vi "UHR-Fleezers Control (fpga) - 11.7.1UCBMeng3RG3(2).vi"() -> ()   [LabVIEW 2014]
doc: "UHR-Fleezers Instrument Control Code (fpga)"
uses:
  <vilib>/Platform/TimedLoop/XDataNode/timing_clust.ctl
  <vilib>/Platform/TimedLoop/XDataNode/nitl_modes.ctl
  <vilib>/Platform/TimedLoop/XDataNode/wakeup.ctl
  <vilib>/rvi/Emulation/niFpgaGetClockAttributes.vi
  <vilib>/rvi/Emulation/niFpgaSctlEmulationGetInTimedLoop.vi
  <vilib>/rvi/Emulation/niFpgaEmulationReportErrorSimple.vi
  <vilib>/rvi/Emulation/niFpgaProcessEmulError.vi
  <vilib>/rvi/eio/common/nirviEmuTemplateMethod_errors.vi
  <vilib>/rvi/Emulation/niFpgaCriticalErrorInLSC.vi
  <vilib>/rvi/interface/RandomDataEmulation/niFpgaRandomDataHandleErrors.vi
  <vilib>/eio/EIONode/EIONode.xnode
  <vilib>/eio/EIOMethodNode/EIOMethodNode.xnode
  <vilib>/rvi/DataTransferAndStorage/Container/XNode/niFpgaContainer.xnode
  <vilib>/rvi/interface/RandomDataEmulation/nirviRandomDataFpgaReadWriteTemplate.vi
  <vilib>/addons/control/pid/fpga.llb/XNode/niFpgaPID.xnode
  <vilib>/Platform/TimedLoop/XDataNode/XDataNode.xnode
  <vilib>/Platform/TimedLoop/XDataNode/XDNodeRunTimeDep.lvlib
panel:
  in  "Tab Control":T1(tab)=enum."Force FB"
  in  "Set 3":bool
  in  "Set 2":bool=TRUE
  in  "Set 1":bool=TRUE
  in  "Trap Pos to FIFO":bool
  in  "N of AI1 Int Acq Sets":i16=2 min=1 max=3 step=1
  out "AI Late Counter":u8
  in  "ai count":u16=400
  in  "+ phase":bool
  in  "Phase count adjustment":i16
  out "Relative phase":i16
  in  "AI to FIFO":bool
  out "BD1 Frequency Out 1":u64
  out "BD1 Frequency Out 2":u64
  out "Trap Pos FIFO Timeout":u16
  out "Trap AI FIFO Timeout":u16
  in  "Trap FIFO Set Timeout":i32
  in  "Tab Control 2":T2(tab)
  in  "FB Offset":u16
  in  "FB Multi Factor":i16
  in  "Dynamic FB (Ronen)":bool
  in  "Negate Intensity FB":bool
  in  "RD":bool
  in  "FB1 output high":i16=3000
  in  "FB1 output low":i16
  in  "D1":i16
  in  "I1":i16=5
  in  "P1":i16=10
  in  "Swap F1 and F2":bool
  in  "Cont. Scan":bool
  in  "Abort scan":bool
  in  "Cycles per step":u64
  in  "Scan BD":bool
  in  "Number of scans":u16
  in  "Scan steps":u64
  in  "Scan freq.  increment":i64
  out "Scanning":bool
  in  "Start scan":bool
  in  "OSK Bd 1":bool
  in  "Reset Bd 1":bool
  in  "PMODE":bool
  in  "Direct RF Box \nCommunication":bool
  in  "Data BD 2":u8 format="%08b"
  in  "Data BD 1":u8 format="%08b"
  in  "Address":u8 format="%02x"
  in  "Update Data":bool
  in  "FPGA Controls\n RF Box":bool
  in  "Number Interlace Cycles":u8=2 min=1 max=3
  in  "Interlace Off Parameters":u8=1 min=1 max=3
  in  "Interlace ON/OFF":bool
  out "DIO Relative phase":i16
  in  "Phase count adjustment (DIO)":i16
  in  "+ phase (DIO)":bool
  out "DIO Late Counter":u8
  in  "DIO count 1 (ticks)":u16=400
  in  "DIO count 2 (ticks)":u16=400
  in  "DIO count 3 (ticks)":u16=400
  out "AI2 Y Sum Set 2":i16
  out "AI2 Y Sum Set 1":i16
  in  "FB Setpoint Set 1":i16 min=0 step=1
  in  "FB Reset Set 1":bool
  in  "FB On/Off Set 1":bool
  in  "FB Reset Set 2":bool
  in  "FB On/Off Set 2":bool
  in  "FB Setpoint Set 2":i16 min=0 step=1
  out "Scan I":u64
  in  "Amp switch delay":u8=5
  in  "XY phase ext loop method":bool
  in  "BD 2 Amplitude 1":u16
  in  "BD 1 Amplitude 1":u16
  in  "BD 2 Frequency 1":u64
  in  "BD 1 Frequency 1":u64
  in  "BD 2 Amplitude 2":u16
  in  "BD 1 Amplitude 2":u16
  in  "BD 2 Frequency 2":u64
  in  "BD 1 Frequency 2":u64
  in  "BD 2 Amplitude 3":u16
  in  "BD 1 Amplitude 3":u16
  in  "BD 2 Frequency 3":u64
  in  "BD 1 Frequency 3":u64
  in  "BD 1 Delay (ticks)":u8
  in  "BD 2 Delay (Ticks)":u8 caption="Count(Ticks)"
  in  "Next trap write delay (ticks)":u8 caption="Count(Ticks)"
  in  "Trap 1 osc enable":bool
  in  "Trap 2 osc enable":bool
  in  "FB Min frequency":u64
  in  "FB Max Frequency":u64
  in  "Dynamic Force FB (Ronen)":bool
  in  "FB2 output high":fxp<+/-,16,1>=0.999969482421875
  in  "FB2 output low":fxp<+/-,16,1>=-1.0
  in  "P2":fxp<+/-,16,8> format="%.11g"
  in  "I2":fxp<+/-,16,8>=10.0 format="%.11g"
  in  "D2":fxp<+/-,16,8> format="%.11g"
  in  "Negate Diff?":bool
  in  "Diff FB Measurement?":bool
  in  "FB Trig Integrate":u32=1
  out "TTrig?":bool
  in  "TTrig Negate Pos":bool=TRUE
  out "Trap Pos FB Int Signal":fxp<+/-,24,9> format="%.18g"
  out "Trap Pos FB Int-Norm Signal":fxp<+/-,16,1> format="%.16g"
  in  "FPGA TTrig Thresh":i64
  in  "FPGA Trap Trig":bool
  out "Trap Pos FB Action":i64
  in  "Trap Pos. FB Offset Factor":i64
  in  "Trap Pos. FB Mult Factor":i64=2
  in  "Trap Pos. FB Reset":bool
  in  "Trap Pos FB Monitor T1 or T2":bool
  in  "AI1 X Scale":u16
  in  "Trap Pos FB Int Count":u16=100
  in  "Trap Pos FB Negate Action":bool
  out "AI1 X Set 2":fxp<+/-,16,1>
  out "AI1 X Set 1":fxp<+/-,16,1>
  in  "Trap Pos. FB SP":fxp<+/-,16,1>
  in  "Force feedback":bool
  out "TTrig Sig":i64
  out "TTrig Fin Thresh":i64
  in  "1D or 2D Scan?":bool
  in  "Abort scan (MCL)":bool
  in  "MCL Scan Axis":bool
  in  "Cont. Scan (MCL)":bool
  out "Scan I (MCL)":u64
  in  "Number of scans (MCL)":u16
  out "Scanning MCL":bool
  in  "Scan steps (MCL)":u64
  in  "Cycles per step (MCL)":u64
  in  "Scan freq.  increment (MCL)":i16
  in  "Start scan (MCL)":bool
  in  "AO2":i16
  in  "AO1":i16
  out "MCL Late Counter":u8
  in  "MCL count":u32=800
  out "MCL Relative Phase":i16
  in  "Phase count adjustment (MCL)":i16
  in  "+ phase (MCL)":bool
  out "APD2 int gate":bool
  out "APD3 out state":bool
  in  "APD Gate Operating Mode":u8 max=2 step=1
  in  "Invert APD Gate":bool
  in  "APD Gate OFF Count":u16=100
  in  "APD Gate ON Count":u16=300
  out "APD 1 Gate Late Counter":u8
  out "APD 1 Gate Relative Phase":i16
  in  "Phase count adjustment (APD 1 Gate)":i16
  in  "+ phase (APD 1 Gate)":bool
  out "APD 2 Counts 0":u32
  out "APD 2 Counts 1":u32
  out "APD 1 Counts 0":u32
  out "APD 1 Counts 1":u32
  out "APD1 out state":bool
  in  "APD AO scale factor":i16=1
  in  "APD to FIFO":bool
  in  "APD Acq Rate Count":u32=20000000
  out "APD Acq Late Counter":u8
  out "APD Acq Relative Phase":i16
  in  "Phase Count Adjustment (APD Acq)":i16
  in  "+ phase (APD Acq)":bool
  in  "Phase count adjustment (APD 2 Gate)":i16
  out "APD 2 Gate Late Counter":u8
  out "APD 2 Gate Relative Phase":i16
  in  "+ phase (APD 2 Gate)":bool
  out "APD2 out state":bool
  out "APD 3 Counts 0":u32
  out "APD 3 Counts 1":u32
  out "APD 3 Gate Late Counter":u8
  in  "Phase count adjustment (APD 3 Gate)":i16
  out "APD 3 Gate Relative Phase":i16
  in  "+ phase (APD 3 Gate)":bool
  out "APD1 int gate":bool
  out "APD3 int gate":bool
  in  "D3":i16
  in  "I3":i16=5
  in  "P3":i16=10
  in  "Green Filter Flipper":bool
  in  "Green FB Count":u16=1200
  out "Green Late Counter":u8
  out "Green FB Relative Phase":i16
  in  "Phase count adjustment (Green FB)":i16=10
  in  "+ phase (Green FB)":bool
  out "Green FB Sum":i16
  in  "Green int current ON count adj":u16=150
  in  "Current Out":u16=30000
  in  "Green FB On/Off":bool
  in  "Green FB Setpoint":i16=250 min=0 step=1
  in  "Green FB Reset":bool
  in  "Operating Mode 2":u8=2 max=2 step=1
  in  "Invert GI 2":bool
  in  "Green interlace OFF count 2":u16=900
  in  "Green interlace ON count 2":u16=300
  out "GI Late Counter 2":u8
  out "GI Relative phase 2":i16
  in  "Phase count adjustment (GI) 2":i16=20
  in  "+ phase (GI) 2":bool
  in  "Green interlace OFF count":u16=100
  out "GI Relative phase":i16
  in  "Phase count adjustment (GI)":i16
  in  "+ phase (GI)":bool
  in  "Green interlace ON count":u16=300
  out "GI Late Counter":u8
  in  "Invert GI":bool
  in  "Operating Mode":u8 max=2 step=1
  in  "+ phase (RI)":bool
  out "RI Relative phase":i16
  out "RI Late Counter":u8
  in  "Red interlace ON count":u16=300
  in  "Red interlace OFF count":u16=100
  in  "Invert RI":bool
  in  "Red Laser Operating Mode":u8 max=2 step=1
  in  "Phase count adjustment (RI)":i16
  out "Red FB Intensity":i16
  in  "RI Current Out":u16=30000
  in  "Red FB On/Off":bool
  in  "D4":i16
  in  "I4":i16=5
  in  "P4":i16=10
  in  "Red FB Setpoint":i16=250 min=0 step=1
  in  "Red FB Reset":bool
  in  "RI Operating Mode 2":u8=2 max=2 step=1
  in  "Invert RI 2":bool
  in  "Phase count adjustment (BI AO)":i16=20
  in  "Blue current ON count adj (AO)":u16=150
  in  "BI Current Out":i16=30000
  in  "Blue FB On/Off":bool
  in  "D5":i16
  in  "I5":i16=5
  in  "P5":i16=10
  in  "Blue FB Setpoint":i16=250 min=0 step=1
  in  "Blue FB Reset":bool
  in  "BI Operating Mode (AO)":u8=2 max=2 step=1
  in  "Invert BI (AO)":bool
  in  "Blue OFF count (AO)":u16=900
  in  "Blue ON count (AO)":u16=300
  out "BI Late Counter (AO)":u8
  out "BI Relative phase (AO)":i16
  in  "+ phase (BI AO)":bool
  in  "Phase count adjustment (BI D)":i16
  in  "Blue Laser Operating Mode (D)":u8 max=2 step=1
  in  "Invert BI (D)":bool
  in  "Blue interlace OFF count (D)":u16=100
  in  "Blue interlace ON count (D)":u16=300
  out "Blue Late Counter (D)":u8
  out "BI Relative phase (D)":i16
  in  "+ phase (BI D)":bool
  out "Blue Intensity":i16
  # "Only one of these can be on\nat a time:"
  # "Raster Scan AOD"
  # "1 (X)"
  # "2 (Y)"
  # "IR Intensity Feedback (RF BD 1)"
  # "FB Gains Set 1"
  # "FB output range 1"
  # "False is usual, True is external loop method"
  # "Parameters if using the external RF switching loop"
  # "Parameters if using the usual internal RF switching method"
  # "FB Triggering Excitation Laser"
  # "Trap Pos. FB Gains"
  # "Trap Pos. FB Range"
  # "AO1 (Y)"
  # "2D"
  # "1D"
  # "AO2 (X)"
  # "APD AO for aligning"
  # "Detection Loop"
  # "Green fluorescent laser digital gate interlacing loop"
  # "0 Forced ON\n1 Forced OFF\n2 Interlacing"
  # "Green FB Gains"
  # "Red fluorescent laser digital gate interlacing loop"
  # "Detection Loop"
  # "0 Forced ON\n1 Forced OFF\n2 Interlacing"
  # "Analog/FB Control Loop\n(Disabled)"
  # "Digital Control Loop"
  # "Blue laser intensity reading"
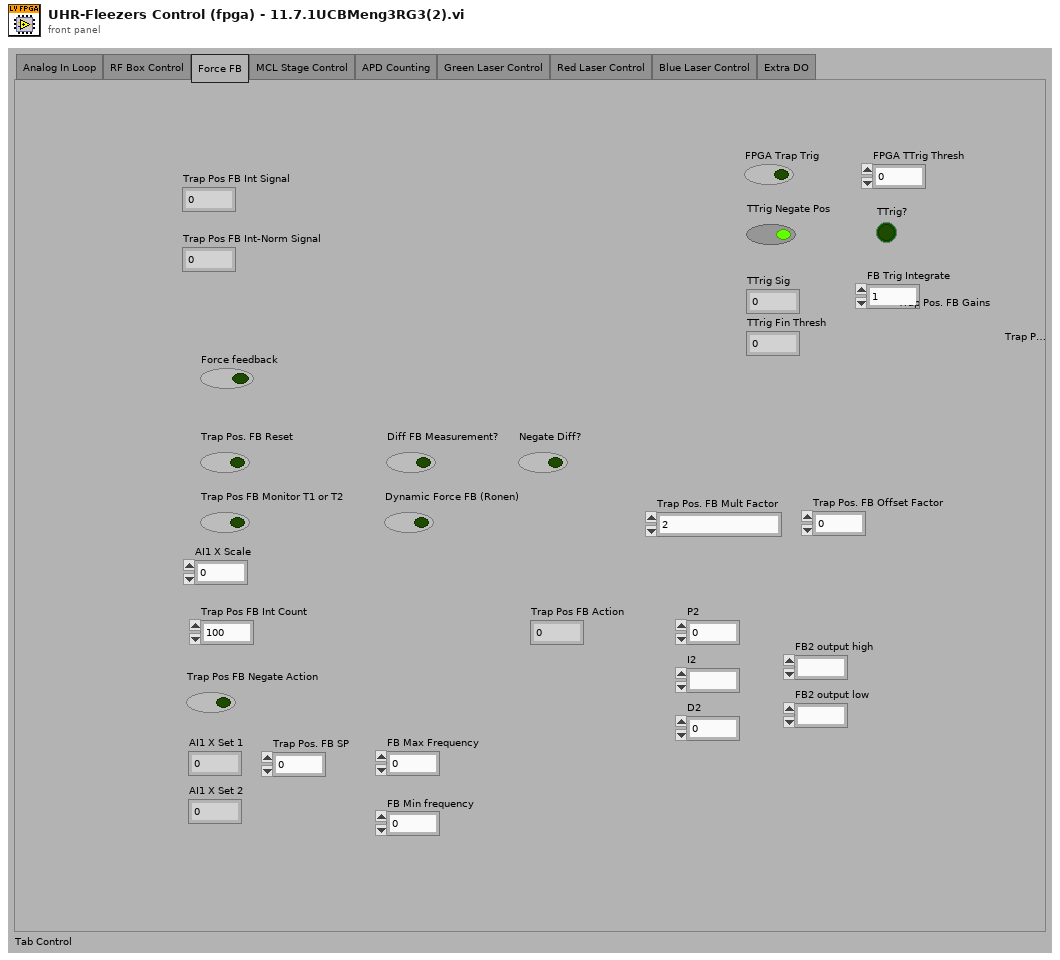
[diagram p1: front panel]
types:
  T1 = enum32{"Analog In Loop", "RF Box Control", "Force FB", "MCL Stage Control", "APD Counting", "Green Laser Control", "Red Laser Control", "Blue Laser Control", "Extra DO"}
  T2 = enum32{"Controls", "Interlacing Frequency and Amplitude Values", "Oscillate trap from memory"}
  T3 = typedef "XDNodeRunTimeDep.lvlib/timing_clust.ctl" = cluster{"Expected End [f-1]":u64, "Actual End [f-1]":u64, "Finished Late? [f-1]":bool, "Expected End [i-1]":u64, "Actual End [i-1]":u64, "Finished Late? [i-1]":bool, "Expected Start [i]":u64, "Actual Start [i]":u64, "Expected Start [f]":u64, "Actual Start [f]":u64, "Source Name":string, "Structure Name":string, "Period":i64, "Deadline":i64, "Offset":i64, "Start":i64, "Priority":i32, "Timeout":i32, "Mode":T4, "Wakeup Reason":T5, "Error":errorcluster, "Source Type":string, "Secondary Source Type":string, "Global End Time":u64, "Global Start Time":u64, "Frame Duration":u64, "Iteration Duration":u64, "Assigned CPU":i32, "I/O Scan Engine Mode":u32}
  T4 = typedef "XDNodeRunTimeDep.lvlib/nitl_modes.ctl" = enum32{"No Change", "Process missed periods, maintain original phase", "Discard missed periods, maintain original phase", "Process missed periods, ignore original phase", "Discard missed periods, ignore original phase"}
  T5 = typedef "XDNodeRunTimeDep.lvlib/wakeup.ctl" = enum32{"Normal", "Aborted", "Asynchronous wakeup", "Timing source error", "Timed loop error", "Timeout"}
  T6 = cluster{"proportional gain (Kc)":i16, "integral gain (Kc*Ts/Ti)":i16, "derivative gain (Kc*Td/Ts)":i16}
  T7 = cluster{"FB1 output high":i16, "FB1 output low":i16}
  T8 = cluster{"P2":fxp<+/-,16,8>, "I2":fxp<+/-,16,8>, "D2":fxp<+/-,16,8>}
  T9 = cluster{"FB2 output high":fxp<+/-,16,1>, "FB2 output low":fxp<+/-,16,1>}
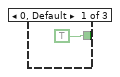
[diagram p2: hidden frame]
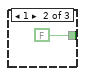
[diagram p3: hidden frame]
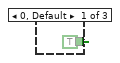
[diagram p4: hidden frame]
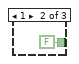
[diagram p5: hidden frame]
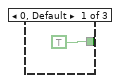
[diagram p7: hidden frame]
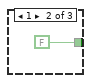
[diagram p8: hidden frame]
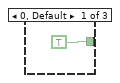
[diagram p10: hidden frame]
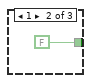
[diagram p11: hidden frame]
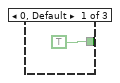
[diagram p14: hidden frame]
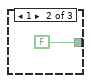
[diagram p15: hidden frame]
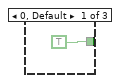
[diagram p17: hidden frame]
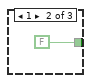
[diagram p18: hidden frame]
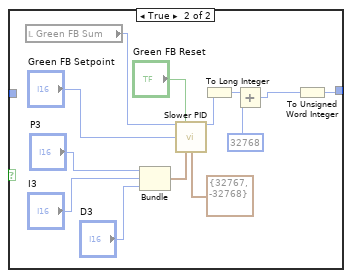
[diagram p20: hidden frame]
diagram:
  w7 = FALSE
  w5 = FALSE
  # "timing array current index"
  # "timing array"
  # "timing counter (phase adjusted here)"
  # "late counter"
  n1 = flat-sequence "FPGA initialization to do before running any of the loops" {
    tunnel: [u16 0 ("DIO count 3 (ticks)")] -> w4
    tunnel: [w15] -> _
    frame #0 {
      w14 = FALSE ("Enable")
      # "BD 2 (Y)"
      # "BD 1 (X)"
      # "Start up expansion chassis early\nto avoid delays later"
      # "This pin controls udclk on the RF boards.\nWhen initially configuring the boards, this pin needs to be\nconfigured as a high impedance input.  Later it will be switched\nto an output."
      # "Initial setting of DIO data and \naddress to low (before reset).  \nThis needs to happen before the other\ncontrol method loops execute."
      n2 = xnode "FPGA I/O Node"("Chassis2/Mod1/AO0"=u16 0 ("Chassis2/Mod4/AO0")) -> ("Chassis2/Mod2/AI0"=w15:i16)  [unwired: 2 in, 2 out]
      n3 = xnode "FPGA I/O Method Node"("Enable"=w14) -> ()  [unwired: 1 in, 1 out]
      n4 = xnode "FPGA I/O Method Node"("Enable"=w14) -> ()  [unwired: 1 in, 1 out]
      n5 = xnode "FPGA I/O Node"("Connector1/DIO0"=FALSE, "Connector1/DIO1"=FALSE, "Connector1/DIO2"=FALSE, "Connector1/DIO3"=FALSE, "Connector1/DIO4"=FALSE, "Connector1/DIO5"=FALSE, "Connector1/DIO6"=FALSE, "Connector1/DIO7"=FALSE, "Connector1/DIO8"=FALSE, "Connector1/DIO9"=FALSE, "Connector1/DIO10"=FALSE, "Connector1/DIO11"=FALSE, "Connector1/DIO12"=FALSE, "Connector1/DIO13"=FALSE, "Connector1/DIO15"=FALSE, "Connector1/DIO20"=FALSE, "Connector1/DIO21"=FALSE, "Connector1/DIO22"=FALSE, "Connector1/DIO23"=FALSE, "Connector1/DIO24"=FALSE, "Connector1/DIO25"=FALSE, "Connector1/DIO26"=FALSE, "Connector1/DIO27"=FALSE, "Connector1/DIO14"=FALSE) -> ()  [unwired: 24 in, 24 out]
    }
  }
  n6 = local read "AO1"() -> (w12:i16)
  n7 = local read "AO2"() -> (w11:i16)
  n8 = node-c288() -> (w10:T3)  [unwired: 1 in]
  n9 = To Unsigned Long Integer(number=w4) -> (unsigned 32bit integer=w8:u32)
  n10 = timed-loop "RF box board DIO control: control bits" {
    timing: w10 -> [_]
    timing-out: [_] -> w9
    tunnel: [w44] -> _
    tunnel: w4 -> [w44]
    stop <- FALSE stop-if-true
    n11 = xnode "FPGA I/O Node"("Connector1/DIO16"="RD", "Connector1/DIO17"="PMODE", "Connector1/DIO18"="OSK Bd 1", "Connector1/DIO19"="Reset Bd 1", "Connector0/DIO3"="Green Filter Flipper") -> ()  [unwired: 5 in, 5 out]
  }
  n12 = disable-structure shown="Disabled" {
    disable-tunnel: w7 -> [w52 _]
    disable-tunnel: w4 -> [w51 _]
    frame Disabled {
      n13 = while "APD 2 Gating" {
        shift-right: [w56] -> _
        shift-left: w51 -> [w61]
        shift-right: [w55] -> _
        shift-left: w52 -> [w53]
        stop <- FALSE stop-if-true
        n14 = flat-sequence {
          tunnel: w61 -> [w64]
          tunnel: [w65] -> w59
          tunnel: [w64] -> w57
          tunnel: [w63] -> w54
          tunnel: w53 -> [w63]
          tunnel: [w68] -> w60
          tunnel: w59 -> [w68]
          tunnel: [w67] -> w58
          tunnel: w57 -> [w67]
          tunnel: w54 -> [w66]
          tunnel: [w90] -> w56
          tunnel: w60 -> [w100]
          tunnel: w58 -> [w98]
          tunnel: [w69] -> w55
          frame #0 {
            n15 = call "Loop Timer8"("Count(Ticks)"=w64) -> ("Tick Count(Ticks)"=w65:u16)
          }
          frame #1 {
            # "Signal maybe then sent through \na transistor before APD"
            n16 = xnode "FPGA I/O Node"("Connector0/DIO8"=w66, "Connector0/DIO9"=w66, "Connector0/DIO10"=w66, "Connector0/DIO11"=w66) -> ()  [unwired: 4 in, 4 out]
            "APD2 int gate" <- w66
          }
          frame #2 {
            n17 = local read "APD Gate ON Count"() -> (w83:u16)
            n18 = local read "APD Gate OFF Count"() -> (w82:u16)
            n19 = feedback #1(TRUE) -> (w95:bool)
            n20 = feedback-in #2(w100) -> ()
            n21 = feedback #2(w100) -> (w84:u16)
            n22 = Not(x=w95) -> (.not. x?=w93:bool)
            n23 = feedback-in #1(w93) -> ()
            n24 = Subtract(x=w100, y=w84) -> (x-y=w99:u16)
            n25 = Select(t=w83, s=w93, f=w82) -> (s? t:f=w97:u16)
            n26 = Subtract(x=w99, y=w98) -> (x-y=w75:u16)
            n27 = Subtract(x=w97, y=w75) -> (x-y=w89:u16)
            n28 = Number To Boolean Array(number=w75) -> (Boolean array=w74:bool[])
            n29 = Or Array Elements(Boolean array=w74) -> (logical OR=w73:bool)
            n30 = Boolean To (0,1)(Boolean="+ phase (APD 2 Gate)") -> (0, 1=w87:i16)
            n31 = Multiply(x=w87, y="Phase count adjustment (APD 2 Gate)") -> (x*y=w85:i16)
            n32 = Boolean To (0,1)(Boolean=w73) -> (0, 1=w80:i16)
            n33 = Add(x=w89, y=w85) -> (x+y=w90:u16)
            n34 = To Unsigned Byte Integer(number=w80) -> (unsigned 8bit integer=w77:u8)
            n35 = feedback #3(i16 0) -> (w92:i16)
            n36 = Subtract(x=w92, y=w85) -> (x-y=w91:i16)
            "APD 2 Gate Relative Phase" <- w91
            n37 = feedback-in #3(w91) -> ()
            n38 = feedback #4(u8 0) -> (w78:u8)
            n39 = Add(x=w77, y=w78) -> (x+y=w76:u8)
            "APD 2 Gate Late Counter" <- w76
            n40 = feedback-in #4(w76) -> ()
            n41 = local read "APD Gate Operating Mode"() -> (w81:u8)
            n42 = case shown="2" w81 {
              tunnel: [TRUE FALSE w103] -> w70
              tunnel: w95 -> [_ _ w103]
              frame 0, Default {
              }
              frame 1 {
              }
              frame 2 {
              }
            }
            n43 = local read "Invert APD Gate"() -> (w72:bool)
            n44 = Not(x=w70) -> (.not. x?=w71:bool)
            n45 = Select(t=w71, s=w72, f=w70) -> (s? t:f=w69:bool)
          }
        }
      }
      n46 = while "APD 1 Gating" {
        shift-right: [w107] -> _
        shift-left: w51 -> [w112]
        shift-right: [w106] -> _
        shift-left: w52 -> [w104]
        stop <- FALSE stop-if-true
        n47 = flat-sequence {
          tunnel: w112 -> [w115]
          tunnel: [w116] -> w110
          tunnel: [w115] -> w108
          tunnel: [w114] -> w105
          tunnel: w104 -> [w114]
          tunnel: [w119] -> w111
          tunnel: w110 -> [w119]
          tunnel: [w118] -> w109
          tunnel: w108 -> [w118]
          tunnel: w105 -> [w117]
          tunnel: [w137] -> w107
          tunnel: w111 -> [w151]
          tunnel: w109 -> [w148]
          tunnel: [w120] -> w106
          frame #0 {
            n48 = call "Loop Timer7"("Count(Ticks)"=w115) -> ("Tick Count(Ticks)"=w116:u16)
          }
          frame #1 {
            # "Signal maybe then sent through \na transistor before APD"
            n49 = xnode "FPGA I/O Node"("Connector0/DIO4"=w117, "Connector0/DIO5"=w117, "Connector0/DIO6"=w117, "Connector0/DIO7"=w117) -> ()  [unwired: 4 in, 4 out]
            "APD1 int gate" <- w117
          }
          frame #2 {
            n50 = feedback #5(TRUE) -> (w143:bool)
            n51 = feedback-in #6(w151) -> ()
            n52 = feedback #6(w151) -> (w150:u16)
            n53 = Not(x=w143) -> (.not. x?=w140:bool)
            n54 = feedback-in #5(w140) -> ()
            n55 = Subtract(x=w151, y=w150) -> (x-y=w149:u16)
            n56 = Select(t="APD Gate ON Count", s=w140, f="APD Gate OFF Count") -> (s? t:f=w145:u16)
            n57 = Subtract(x=w149, y=w148) -> (x-y=w125:u16)
            n58 = Subtract(x=w145, y=w125) -> (x-y=w136:u16)
            n59 = Number To Boolean Array(number=w125) -> (Boolean array=w126:bool[])
            n60 = Or Array Elements(Boolean array=w126) -> (logical OR=w124:bool)
            n61 = Boolean To (0,1)(Boolean="+ phase (APD 1 Gate)") -> (0, 1=w134:i16)
            n62 = Boolean To (0,1)(Boolean=w124) -> (0, 1=w131:i16)
            n63 = Multiply(x=w134, y="Phase count adjustment (APD 1 Gate)") -> (x*y=w132:i16)
            n64 = To Unsigned Byte Integer(number=w131) -> (unsigned 8bit integer=w128:u8)
            n65 = Add(x=w136, y=w132) -> (x+y=w137:u16)
            n66 = feedback #7(i16 0) -> (w139:i16)
            n67 = Subtract(x=w139, y=w132) -> (x-y=w138:i16)
            "APD 1 Gate Relative Phase" <- w138
            n68 = feedback-in #7(w138) -> ()
            n69 = feedback #8(u8 0) -> (w129:u8)
            n70 = Add(x=w128, y=w129) -> (x+y=w127:u8)
            "APD 1 Gate Late Counter" <- w127
            n71 = feedback-in #8(w127) -> ()
            n72 = case shown="2" "APD Gate Operating Mode" {
              tunnel: [TRUE FALSE w154] -> w121
              tunnel: w143 -> [_ _ w154]
              frame 0, Default {
              }
              frame 1 {
              }
              frame 2 {
              }
            }
            n73 = Not(x=w121) -> (.not. x?=w122:bool)
            n74 = Select(t=w122, s="Invert APD Gate", f=w121) -> (s? t:f=w120:bool)
          }
        }
      }
    }
    frame Enabled {
    }
  }
  n75 = while "RF box board direct communication loop" {
    tunnel: w4 -> [_]
    stop <- FALSE stop-if-true
    n76 = case "Whether to use direct communication method (only use one method at a time)" shown="True" "Direct RF Box \nCommunication" {
      frame False {
      }
      frame True {
        n77 = case shown="True" "Update Data" {
          frame False {
          }
          frame True {
            n78 = flat-sequence {
              frame #0 {
                n79 = First Call?() -> (First Call?: T/F=w158:bool)
                n80 = case shown="True" w158 {
                  frame False {
                  }
                  frame True {
                    # "If first time data updated, be sure to set WR high\nbefore setting data and address bits."
                    n81 = flat-sequence {
                      frame #0 {
                        n82 = xnode "FPGA I/O Node"("Connector1/DIO15"=TRUE) -> ()  [unwired: 1 in, 1 out]
                      }
                      frame #1 {
                        n83 = call "Wait"("Count(Ticks)"=u8 40 ("DO Delay 3 (Ticks)")) -> ()  [unwired: 1 out]
                      }
                    }
                  }
                }
              }
              frame #1 {
                n84 = Number To Boolean Array(number="Address") -> (Boolean array=w207:bool[])
                n85 = Number To Boolean Array(number="Data BD 1") -> (Boolean array=w208:bool[])
                n86 = Number To Boolean Array(number="Data BD 2") -> (Boolean array=w177:bool[])
                n87 = Index Array(array=w208, index=7) -> (element=w192:bool)
                n88 = Index Array(array=w208, index=6) -> (element=w191:bool)
                n89 = Index Array(array=w208, index=5) -> (element=w190:bool)
                n90 = Index Array(array=w208, index=4) -> (element=w189:bool)
                n91 = Index Array(array=w208, index=3) -> (element=w188:bool)
                n92 = Index Array(array=w208, index=2) -> (element=w187:bool)
                n93 = Index Array(array=w208, index=1) -> (element=w186:bool)
                n94 = Index Array(array=w208, index=0) -> (element=w185:bool)
                n95 = Index Array(array=w207, index=5) -> (element=w184:bool)
                n96 = Index Array(array=w207, index=4) -> (element=w183:bool)
                n97 = Index Array(array=w207, index=3) -> (element=w182:bool)
                n98 = Index Array(array=w207, index=2) -> (element=w181:bool)
                n99 = Index Array(array=w207, index=1) -> (element=w180:bool)
                n100 = Index Array(array=w207, index=0) -> (element=w179:bool)
                n101 = Index Array(array=w177, index=7) -> (element=w168:bool)
                n102 = Index Array(array=w177, index=6) -> (element=w167:bool)
                n103 = Index Array(array=w177, index=5) -> (element=w166:bool)
                n104 = Index Array(array=w177, index=4) -> (element=w165:bool)
                n105 = Index Array(array=w177, index=3) -> (element=w164:bool)
                n106 = Index Array(array=w177, index=2) -> (element=w163:bool)
                n107 = Index Array(array=w177, index=1) -> (element=w162:bool)
                n108 = Index Array(array=w177, index=0) -> (element=w161:bool)
                n109 = xnode "FPGA I/O Node"("Connector1/DIO0"=w192, "Connector1/DIO1"=w191, "Connector1/DIO2"=w190, "Connector1/DIO3"=w189, "Connector1/DIO4"=w188, "Connector1/DIO5"=w187, "Connector1/DIO6"=w186, "Connector1/DIO7"=w185, "Connector1/DIO8"=w184, "Connector1/DIO9"=w183, "Connector1/DIO10"=w182, "Connector1/DIO11"=w181, "Connector1/DIO12"=w180, "Connector1/DIO13"=w179, "Connector1/DIO20"=w168, "Connector1/DIO21"=w167, "Connector1/DIO22"=w166, "Connector1/DIO23"=w165, "Connector1/DIO24"=w164, "Connector1/DIO25"=w163, "Connector1/DIO26"=w162, "Connector1/DIO27"=w161) -> ()  [unwired: 22 in, 22 out]
              }
              frame #2 {
                # "wait and then apply write signal"
                n110 = call "Wait2"("Count(Ticks)"=u8 40 ("DO Delay 1 (Ticks)")) -> ()  [unwired: 1 out]
              }
              frame #3 {
                # "sending bit low writes data to board buffer"
                n111 = xnode "FPGA I/O Node"("Connector1/DIO15"=FALSE) -> ()  [unwired: 1 in, 1 out]
              }
              frame #4 {
                # "wait then return write signal"
                n112 = call "Wait3"("Count(Ticks)"=u8 40 ("DO Delay 2 (Ticks)")) -> ()  [unwired: 1 out]
              }
              frame #5 {
                # "sending bit high makes ready to\nwrite more data"
                n113 = xnode "FPGA I/O Node"("Connector1/DIO15"=TRUE) -> ()  [unwired: 1 in, 1 out]
              }
            }
          }
        }
      }
    }
  }
  n114 = while "RF box board DIO control: parallel communication" {
    shift-right: [w227] -> _
    shift-left: w4 -> [w226]
    shift-right: [w225] -> _
    shift-left: FALSE ("Swap F1 and F2") -> [w224]
    shift-right: [w219] -> _
    shift-left: u16 0 -> [w220]
    shift-right: [w217] -> _
    shift-left: u16 0 -> [w218]
    shift-right: [w215] -> _
    shift-left: u64 0 -> [w216]
    stop <- FALSE stop-if-true
    n115 = flat-sequence {
      tunnel: w224 -> [w231]
      tunnel: w226 -> [w229]
      tunnel: [w231] -> w223
      tunnel: [w230] -> w222
      tunnel: [w229] -> w221
      tunnel: [w243] -> w227
      tunnel: [w242] -> w225
      tunnel: w223 -> [w241]
      tunnel: w222 -> [w239]
      tunnel: w221 -> [w238]
      tunnel: w220 -> [w237]
      tunnel: [w236] -> w219
      tunnel: w218 -> [w235]
      tunnel: [w234] -> w217
      tunnel: w216 -> [w233]
      tunnel: [w232] -> w215
      frame #0 {
        n116 = call "Loop Timer"("Count(Ticks)"=w229) -> ("Tick Count(Ticks)"=w230:u16)
      }
      frame #1 {
        n117 = flat-sequence {
          tunnel: ["FPGA Controls\n RF Box"] -> w240
          tunnel: w241 -> [w244]
          tunnel: [w307] -> w243
          tunnel: [w320] -> w242
          tunnel: w240 -> [w319]
          tunnel: w239 -> [w313]
          tunnel: w238 -> [w310]
          tunnel: w237 -> [w276]
          tunnel: [w275] -> w236
          tunnel: w235 -> [w272]
          tunnel: [w271] -> w234
          tunnel: w233 -> [w270]
          tunnel: [w269] -> w232
          frame #0 {
            n118 = case shown="True" "FPGA Controls\n RF Box" {
              tunnel: w244 -> [_ w246]
              frame False {
              }
              frame True {
                n119 = flat-sequence {
                  tunnel: w246 -> [w256]
                  frame #0 {
                    n120 = First Call?() -> (First Call?: T/F=w247:bool)
                    n121 = case shown="True" w247 {
                      frame False {
                      }
                      frame True {
                        # "BD 2"
                        # "BD 1"
                        # "If first time data updated, be sure to set WR high and UDCLK low\nbefore setting data and address bits."
                        n122 = xnode "FPGA I/O Method Node"("Enable"=TRUE) -> ("FPGA I/O Out"=w249:refnum<k21>)  [unwired: 1 in]
                        n123 = xnode "FPGA I/O Method Node"("Enable"=TRUE) -> ("FPGA I/O Out"=w252:refnum<k21>)  [unwired: 1 in]
                        n124 = xnode "FPGA I/O Node"("Connector1/DIO15"=TRUE) -> ()  [unwired: 1 in, 1 out]
                        n125 = xnode "FPGA I/O Node"("I/O Item"=FALSE ("Connector1/DIO30"), "FPGA I/O In"=w249) -> ()  [unwired: 1 out]
                        n126 = xnode "FPGA I/O Node"("I/O Item"=FALSE ("Connector1/DIO30"), "FPGA I/O In"=w252) -> ()  [unwired: 1 out]
                      }
                    }
                  }
                  frame #1 {
                    n127 = case shown="False" FALSE {
                      tunnel: w256 -> [w258 _]
                      frame False {
                        # "Usual operation"
                        n128 = flat-sequence "BD 1 (X)" {
                          tunnel: w258 -> [w265]
                          tunnel: "Amp switch delay" -> [w266]
                          frame #0 {
                            n129 = call "Wait6"("Count(Ticks)"="BD 1 Delay (ticks)") -> ()  [unwired: 1 out]
                          }
                          frame #1 {
                            # "switch frequency"
                            n130 = xnode "FPGA I/O Node"("Connector1/DIO36"=w265) -> ()  [unwired: 1 in, 1 out]
                          }
                          frame #2 {
                            # "~5 ticks is usual"
                            n131 = call "Wait4"("Count(Ticks)"=w266) -> ()  [unwired: 1 out]
                          }
                          frame #3 {
                            # "this switches amplitude"
                            # "switch amplitude"
                            # "send udclk high"
                            n132 = xnode "FPGA I/O Node"("Connector1/DIO30"=TRUE ("Connector1/DIO15")) -> ()  [unwired: 1 in, 1 out]
                          }
                          frame #4 {
                            # "reset to be ready for next\ncycle"
                            # "send udclk low"
                            n133 = xnode "FPGA I/O Node"("Connector1/DIO30"=FALSE ("Connector1/DIO15")) -> ()  [unwired: 1 in, 1 out]
                          }
                        }
                        n134 = flat-sequence "BD 2 (Y)" {
                          tunnel: w258 -> [w260]
                          tunnel: "Amp switch delay" -> [w261]
                          frame #0 {
                            n135 = call "Wait7"("Count(Ticks)"="BD 2 Delay (Ticks)") -> ()  [unwired: 1 out]
                          }
                          frame #1 {
                            # "switch frequency"
                            n136 = xnode "FPGA I/O Node"("Connector1/DIO37"=w260) -> ()  [unwired: 1 in, 1 out]
                          }
                          frame #2 {
                            # "~5 ticks is usual"
                            n137 = call "Wait5"("Count(Ticks)"=w261) -> ()  [unwired: 1 out]
                          }
                          frame #3 {
                            # "this switches amplitude"
                            # "switch amplitude"
                            # "send udclk high"
                            n138 = xnode "FPGA I/O Node"("Connector1/DIO29"=TRUE ("Connector1/DIO15")) -> ()  [unwired: 1 in, 1 out]
                          }
                          frame #4 {
                            # "reset to be ready for next\ncycle"
                            # "send udclk low"
                            n139 = xnode "FPGA I/O Node"("Connector1/DIO29"=FALSE ("Connector1/DIO15")) -> ()  [unwired: 1 in, 1 out]
                          }
                        }
                      }
                      frame True {
                        # "Operation when you need a long delay for either X or Y to synchonize AOD light out phase (> ~100 ticks)."
                        # "Trigger the external loop by sending the boolean FSK value through a FIFO"
                      }
                    }
                  }
                }
              }
            }
          }
          frame #1 {
            # "This is the prior cycle's on time"
            # "increment timing\nindex, reset to 0 if \nend of matrix"
            # "Reset to begginning (1) when number of cycles reached."
            # "timing index"
            # "build byte stacks for writing data\n(must correspond to addresses array constant)"
            # "Timing housekeeping"
            # "Adjust phase if late\n(maintains constant phase relationship between cycles)"
            n140 = Bundle("FB1 output high"="FB1 output high", "FB1 output low"="FB1 output low") -> (w280:T7)  [unwired: 1 in]
            n141 = Bundle("P1"="P1", "I1"="I1", "D1"="D1") -> (w281:cluster{"P1":i16, "I1":i16, "D1":i16})  [unwired: 1 in]
            n142 = feedback #9(u8 0 ("t")) -> (w316:u8)
            n143 = Increment(x=w316) -> (x+1=w359:u8)
            n144 = Increment(x="Number Interlace Cycles") -> (x+1=w354:u8)
            n145 = Equal?(x=w359, y=w354) -> (x = y?=w361:bool)
            n146 = Select(t=u8 1, s=w361, f=w359) -> (s? t:f=w315:u8)
            n147 = feedback-in #9(w315) -> ()
            n148 = Increment(x=w315) -> (x+1=w356:u8)
            n149 = Equal?(x=w356, y=w354) -> (x = y?=w357:bool)
            n150 = Select(t=u8 1, s=w357, f=w356) -> (s? t:f=w353:u8)
            n151 = Select(t=w353, s="Interlace ON/OFF", f="Interlace Off Parameters") -> (s? t:f=w279:u8)
            n152 = case shown="1, Default" w279 {
              tunnel: [w400 w655 "BD 1 Frequency 3"] -> w349
              tunnel: [w450 "BD 2 Frequency 2" "BD 2 Frequency 3"] -> w338
              tunnel: ["BD 2 Amplitude 1" "BD 2 Amplitude 2" "BD 2 Amplitude 3"] -> w295
              tunnel: [w409 w649 "BD 1 Amplitude 3"] -> w298
              tunnel: w281 -> [w417 w657 _]
              tunnel: w280 -> [w418 w656 _]
              tunnel: "Negate Intensity FB" -> [w416 w653 _]
              tunnel: "Dynamic FB (Ronen)" -> [w415 w652 _]
              tunnel: w276 -> [w410 w651 w703]
              tunnel: [w409 w651 w703] -> w275
              tunnel: "FB Multi Factor" -> [w408 w648 _]
              tunnel: "FB Offset" -> [w407 w647 _]
              tunnel: w272 -> [w406 w650 w702]
              tunnel: [w406 w649 w702] -> w271
              tunnel: w270 -> [w405 w646 w701]
              tunnel: [w400 w646 w701] -> w269
              frame 1, Default {
                w433 = fxp<+/-,24,9> 0.0 ("AI1 X Set 2")
                w426 = u16 0
                w446 = u64 0 ("f")
                # "Added by Ronen -\nUpper and Lower \nLimits for the FB \ngenerated frequency\nto avoid losing bead \nwhen tether breaks"
                # "Changed by Ronen - correction \nby PID is now implemented not on \nthe Base BD1 frequency but on the last\nfrequency sent."
                # "BD1 Amp 1"
                # "Changed by Ronen-\n FB changed \nso that value from PID is added to\nlast amplitude sent to board. Correction\nValue can be scaled down same as the force\nFB value."
                # "This signal integration happens no matter what\nso that correct setpoints can be chosen before \nturning on the FB."
                # "Trap 1"
                n153 = local read "AI1 X Set 2"() -> (w429:fxp<+/-,16,1>)
                n154 = local read "AI1 X Set 1"() -> (w430:fxp<+/-,16,1>)
                n155 = local read "Scanning"() -> (w451:bool)
                n156 = Or(x=w451, y="Start scan") -> (x .or. y?=w444:bool)
                n157 = case shown="True" "Diff FB Measurement?" {
                  tunnel: w429 -> [w469 w478]
                  tunnel: w430 -> [w468 w479]
                  tunnel: [w466 w470] -> w431
                  frame False {
                    n158 = Select(t=w468, s="Trap Pos FB Monitor T1 or T2", f=w469) -> (s? t:f=w466:fxp<+/-,16,1>)
                  }
                  frame True {
                    n159 = Subtract(x=w479, y=w478) -> (x-y=w471:fxp<+/-,17,2>)
                    n160 = Not(x="Negate Diff?") -> (.not. x?=w477:bool)
                    n161 = Boolean To (0,1)(Boolean="Negate Diff?") -> (0, 1=w475:i16)
                    n162 = Boolean To (0,1)(Boolean=w477) -> (0, 1=w476:i16)
                    n163 = Negate(x=w475) -> (-x=w474:i16)
                    n164 = Add(x=w474, y=w476) -> (x+y=w472:i16)
                    n165 = Multiply(x=w472, y=w471) -> (x*y=w470:fxp<+/-,32,17>)
                  }
                }
                n166 = Not(x="Abort scan") -> (.not. x?=w442:bool)
                n167 = And(x=w442, y=w444) -> (x .and. y?=w441:bool)
                n168 = case "For raster scanning" shown="False" w441 {
                  tunnel: [u64 0 w605] -> w447
                  tunnel: "Start scan" -> [_ w590]
                  frame False {
                    n169 = local write "Scanning"(FALSE ("scanning")) -> ()
                  }
                  frame True {
                    w574 = i64 0
                    w573 = u64 0
                    # "scan incr."
                    # "freq. incr. mult."
                    # "count steps"
                    # "count number of cycles"
                    n170 = feedback #10(w573) -> (w602:u64)
                    n171 = Select(t=w573, s=w590, f=w602) -> (s? t:f=w604:u64)
                    n172 = Increment(x=w604) -> (x+1=w601:u64)
                    n173 = Greater?(x="Cycles per step", y=w601) -> (0:w583:bool)
                    n174 = Select(t=w601, s=w583, f=w573) -> (s? t:f=w600:u64)
                    n175 = feedback-in #10(w600) -> ()
                    n176 = feedback #11(w573) -> (w599:u64)
                    n177 = Select(t=w573, s=w590, f=w599) -> (s? t:f=w594:u64)
                    n178 = Increment(x=w594) -> (x+1=w598:u64)
                    n179 = Add(x="Scan steps", y="Scan steps") -> (x+y=w597:u64)
                    n180 = Select(t=w594, s=w583, f=w598) -> (s? t:f=w578:u64)
                    n181 = Greater?(x=w597, y=w578) -> (0:w577:bool)
                    n182 = Select(t=w578, s=w577, f=w573) -> (s? t:f=w595:u64)
                    n183 = feedback-in #11(w595) -> ()
                    n184 = Equal?(x="Scan steps", y=w578) -> (x = y?=w582:bool)
                    n185 = Greater?(x="Scan steps", y=w594) -> (0:w593:bool)
                    n186 = feedback #12(w574) -> (w596:i64)
                    n187 = Select(t=w574, s=w590, f=w596) -> (s? t:f=w580:i64)
                    n188 = Increment(x=w580) -> (x+1=w592:i64)
                    n189 = Decrement(x=w580) -> (x-1=w591:i64)
                    n190 = Select(t=w592, s=w593, f=w591) -> (s? t:f=w581:i64)
                    n191 = Select(t=w580, s=w582, f=w581) -> (s? t:f=w579:i64)
                    n192 = Select(t=w580, s=w583, f=w579) -> (s? t:f=w575:i64)
                    n193 = Select(t=w575, s=w577, f=w574) -> (s? t:f=w576:i64)
                    n194 = feedback-in #12(w576) -> ()
                    n195 = feedback #13(w573) -> (w589:u64)
                    n196 = Select(t=w573, s=w590, f=w589) -> (s? t:f=w585:u64)
                    n197 = Increment(x=w585) -> (x+1=w586:u64)
                    n198 = Select(t=w585, s=w577, f=w586) -> (s? t:f=w584:u64)
                    n199 = Greater?(x="Number of scans", y=w584) -> (0:w570:bool)
                    n200 = Multiply(x="Scan freq.  increment", y=w580) -> (x*y=w605:i64)
                    n201 = Select(t=TRUE, s="Cont. Scan", f=w570) -> (s? t:f=w569:bool)
                    "Scanning" <- w569
                    n202 = Select(t=w584, s=w569, f=w573) -> (s? t:f=w587:u64)
                    n203 = feedback-in #13(w587) -> ()
                    n204 = Increment(x=w584) -> (x+1=→"Scan I":u64)
                  }
                }
                n205 = feedback #14(w426) -> (w425:u16)
                n206 = Increment(x=w425) -> (x+1=w427:u16)
                n207 = Greater Or Equal?(x=w427, y="Trap Pos FB Int Count") -> (x >= y?=w404:bool)
                n208 = Select(t=w426, s=w404, f=w427) -> (s? t:f=w428:u16)
                n209 = feedback-in #14(w428) -> ()
                n210 = feedback #15(w433) -> (w432:fxp<+/-,24,9>)
                n211 = Add(x=w431, y=w432) -> (x+y=w424:fxp<+/-,24,9>)
                n212 = case "For intensity feedback" shown="True" "FB On/Off Set 1" {
                  tunnel: w410 -> [_ w610]
                  tunnel: ["BD 1 Amplitude 1" w616] -> w409
                  tunnel: w418 -> [_ w617]
                  tunnel: w417 -> [_ w618]
                  tunnel: w416 -> [_ w615]
                  tunnel: w415 -> [_ w614]
                  tunnel: w408 -> [_ w609]
                  tunnel: w407 -> [_ w608]
                  frame False {
                  }
                  frame True {
                    n213 = local read "AI2 Y Sum Set 1"() -> (w612:i16)
                    n214 = case shown="True" w614 {
                      tunnel: w618 -> [w624 w638]
                      tunnel: w617 -> [w625 w637]
                      tunnel: [w619 w636] -> w616
                      tunnel: w615 -> [_ w635]
                      tunnel: "FB Setpoint Set 1" -> [w623 w634]
                      tunnel: w612 -> [w622 w633]
                      tunnel: "FB Reset Set 1" -> [w621 w632]
                      tunnel: w610 -> [_ w631]
                      tunnel: w609 -> [_ w629]
                      tunnel: w608 -> [_ w627]
                      frame False {
                        n215 = call "Slower PID.vi"("process variable"=w622, "reset?"=w621, "setpoint"=w623, "PID gains (x 2^8)"=w624, "output range"=w625) -> ("output"=w620:i16)  [unwired: 10 out]
                        n216 = To Unsigned Word Integer(number=w620) -> (unsigned 16bit integer=w619:u16)
                      }
                      frame True {
                        n217 = call "Slower PID.vi"("process variable"=w633, "reset?"=w632, "setpoint"=w634, "PID gains (x 2^8)"=w638, "output range"=w637) -> ("output"=w639:i16)  [unwired: 10 out]
                        n218 = To Unsigned Word Integer(number=w639) -> (unsigned 16bit integer=w630:u16)
                        n219 = Scale By Power Of 2(n=w629, x=w630) -> (x*2^n=w628:u16)
                        n220 = Add(x=w628, y=w627) -> (x+y=w626:u16)
                        n221 = case shown="True" w635 {
                          tunnel: w626 -> [w642 w644]
                          tunnel: w631 -> [w640 w645]
                          tunnel: [w641 w643] -> w636
                          frame False {
                            n222 = Add(x=w640, y=w642) -> (x+y=w641:u16)
                          }
                          frame True {
                            n223 = Subtract(x=w645, y=w644) -> (x-y=w643:u16)
                          }
                        }
                      }
                    }
                  }
                }
                n224 = Select(t=w433, s=w404, f=w424) -> (s? t:f=w436:fxp<+/-,24,9>)
                n225 = feedback-in #15(w436) -> ()
                n226 = Divide(x=w424, y="Trap Pos FB Int Count") -> (x/y=w419:fxp<+/-,16,1>)
                n227 = feedback #16(fxp<+/-,24,9> 0.0 ("AI1 X Set 2")) -> (w437:fxp<+/-,24,9>)
                n228 = Select(t=w424, s=w404, f=w437) -> (s? t:f=w438:fxp<+/-,24,9>)
                "Trap Pos FB Int Signal" <- w438
                n229 = feedback-in #16(w438) -> ()
                n230 = feedback #17(fxp<+/-,16,1> 0.0 ("Trap Pos FB Int-Norm Signal")) -> (w421:fxp<+/-,16,1>)
                n231 = Select(t=w419, s=w404, f=w421) -> (s? t:f=w420:fxp<+/-,16,1>)
                "Trap Pos FB Int-Norm Signal" <- w420
                n232 = feedback-in #17(w420) -> ()
                n233 = case "For position feedback" shown="True" "Force feedback" {
                  tunnel: [i64 0 w485] -> w414
                  tunnel: w419 -> [_ w482]
                  tunnel: w404 -> [_ w481]
                  frame False {
                  }
                  frame True {
                    n234 = feedback #18(i64 0) -> (w484:i64)
                    n235 = case shown="False" w481 {
                      tunnel: [w486 w500] -> w485
                      tunnel: w484 -> [w486 _]
                      tunnel: w482 -> [_ w494]
                      frame False {
                      }
                      frame True {
                        w504 = u32 0
                        n236 = Bundle("P2"="P2", "I2"="I2", "D2"="D2") -> (w490:T8)  [unwired: 1 in]
                        n237 = Bundle("FB2 output high"="FB2 output high", "FB2 output low"="FB2 output low") -> (w487:T9)  [unwired: 1 in]
                        n238 = xnode ("PID")("process variable"=w494, "reset?"="Trap Pos. FB Reset", "setpoint"="Trap Pos. FB SP", "PID gains"=w490, "output range"=w487) -> ("output"=w516:fxp<+/-,16,1>)
                        n239 = Negate(x=w516) -> (-x=w515:fxp<+/-,17,2>)
                        n240 = Select(t=w515, s="Trap Pos FB Negate Action", f=w516) -> (s? t:f=w512:fxp<+/-,17,2>)
                        n241 = Scale By Power Of 2(n=u32 15, x=u32 1) -> (x*2^n=w509:u32)
                        n242 = Multiply(x=w512, y=w509) -> (x*y=w508:fxp<+/-,17,17>)
                        n243 = To Quad Integer(1:w508) -> (0:w520:i64)
                        "Trap Pos FB Action" <- w520
                        n244 = Multiply(x=w520, y="Trap Pos. FB Mult Factor") -> (x*y=w518:i64)
                        n245 = Add(x=w518, y="Trap Pos. FB Offset Factor") -> (x+y=w500:i64)
                        n246 = feedback #19() -> (w501:i64)  [unwired: 1 in]
                        n247 = Add(x=w500, y=w501) -> (x+y=w498:i64)
                        n248 = feedback #20(w504) -> (w506:u32)
                        n249 = Increment(x=w506) -> (x+1=w495:u32)
                        n250 = Greater Or Equal?(x=w495, y="FB Trig Integrate") -> (x >= y?=w496:bool)
                        n251 = Select(t=i64 0, s=w496, f=w498) -> (s? t:f=w502:i64)
                        n252 = feedback-in #19(w502) -> ()
                        n253 = Select(t=w504, s=w496, f=w495) -> (s? t:f=w505:u32)
                        n254 = feedback-in #20(w505) -> ()
                        n255 = And(x=w496, y="FPGA Trap Trig") -> (x .and. y?=w503:bool)
                        n256 = case "Trap FB trigger excitation laser ON" shown="True" w503 {
                          tunnel: w498 -> [_ w524]
                          tunnel: w495 -> [_ w522]
                          frame False {
                          }
                          frame True {
                            n257 = Not(x="TTrig Negate Pos") -> (.not. x?=w531:bool)
                            n258 = Boolean To (0,1)(Boolean="TTrig Negate Pos") -> (0, 1=w529:i16)
                            n259 = Boolean To (0,1)(Boolean=w531) -> (0, 1=w530:i16)
                            n260 = Negate(x=w529) -> (-x=w528:i16)
                            n261 = Add(x=w528, y=w530) -> (x+y=w527:i16)
                            n262 = Multiply(x=w527, y=w524) -> (x*y=w526:i64)
                            "TTrig Sig" <- w526
                            n263 = Multiply(x="FPGA TTrig Thresh", y=w522) -> (x*y=w523:i64)
                            "TTrig Fin Thresh" <- w523
                            n264 = Greater Or Equal?(x=w526, y=w523) -> (x >= y?=w525:bool)
                            n265 = case shown="True" w525 {
                              frame False {
                              }
                              frame True {
                                w534 = TRUE ("Green FB On/Off")
                                w536 = u8 2 ("Operating Mode")
                                n266 = local write "Operating Mode 2"(w536) -> ()
                                n267 = local write "Operating Mode"(w536) -> ()
                                n268 = local write "Green FB On/Off"(w534) -> ()
                                n269 = local write "FPGA Trap Trig"(FALSE ("FPGA Trap Trig")) -> ()
                                "TTrig?" <- w534
                              }
                            }
                          }
                        }
                      }
                    }
                    n270 = feedback-in #18(w485) -> ()
                  }
                }
                n271 = case shown="True" "Dynamic Force FB (Ronen)" {
                  tunnel: w414 -> [w457 w461]
                  tunnel: [w456 w460] -> w412
                  tunnel: w405 -> [_ w459]
                  tunnel: w404 -> [_ w458]
                  frame False {
                    # "(BD1 Frequency 1)"
                    n272 = Add(x="BD 1 Frequency 1", y=w457) -> (x+y=w456:u64)
                  }
                  frame True {
                    n273 = case shown="True" w458 {
                      tunnel: w461 -> [_ w465]
                      tunnel: [w462 w464] -> w460
                      tunnel: w459 -> [w462 w463]
                      frame False {
                      }
                      frame True {
                        n274 = Add(x=w463, y=w465) -> (x+y=w464:u64)
                      }
                    }
                  }
                }
                n275 = Select(t=w446, s="Scan BD", f=w447) -> (s? t:f=w445:u64)
                n276 = Select(t=w447, s="Scan BD", f=w446) -> (s? t:f=w448:u64)
                n277 = Add(x=w445, y="BD 2 Frequency 1") -> (x+y=w450:u64)
                n278 = Compound Arithmetic op=ADD(i64 0 ("f"), w412, w448) -> (w403:u64)
                "BD1 Frequency Out 1" <- w403
                n279 = In Range and Coerce(upper limit="FB Max Frequency", x=w403, lower limit="FB Min frequency") -> (coerced(x)=w400:u64)  [unwired: 1 out]
              }
              frame 2 {
                # "Trap 2"
                n280 = case shown="True" "FB On/Off Set 2" {
                  tunnel: ["BD 1 Amplitude 2" w667] -> w649
                  tunnel: w650 -> [_ w665]
                  tunnel: w657 -> [_ w670]
                  tunnel: w656 -> [_ w669]
                  tunnel: w653 -> [_ w668]
                  tunnel: w652 -> [_ w666]
                  tunnel: w648 -> [_ w664]
                  tunnel: w647 -> [_ w663]
                  frame False {
                  }
                  frame True {
                    n281 = local read "AI2 Y Sum Set 2"() -> (w672:i16)
                    n282 = case shown="False" w666 {
                      tunnel: "FB Setpoint Set 2" -> [w678 w694]
                      tunnel: w672 -> [w679 w693]
                      tunnel: "FB Reset Set 2" -> [w680 w692]
                      tunnel: w670 -> [w676 w690]
                      tunnel: w669 -> [w677 w689]
                      tunnel: w668 -> [_ w688]
                      tunnel: [w674 w687] -> w667
                      tunnel: w665 -> [_ w686]
                      tunnel: w664 -> [_ w685]
                      tunnel: w663 -> [_ w682]
                      frame False {
                        n283 = call "Slower PID.vi"("process variable"=w679, "reset?"=w680, "setpoint"=w678, "PID gains (x 2^8)"=w676, "output range"=w677) -> ("output"=w675:i16)  [unwired: 10 out]
                        n284 = To Unsigned Word Integer(number=w675) -> (unsigned 16bit integer=w674:u16)
                      }
                      frame True {
                        n285 = call "Slower PID.vi"("process variable"=w693, "reset?"=w692, "setpoint"=w694, "PID gains (x 2^8)"=w690, "output range"=w689) -> ("output"=w691:i16)  [unwired: 10 out]
                        n286 = To Unsigned Word Integer(number=w691) -> (unsigned 16bit integer=w684:u16)
                        n287 = Scale By Power Of 2(n=w685, x=w684) -> (x*2^n=w683:u16)
                        n288 = Add(x=w683, y=w682) -> (x+y=w681:u16)
                        n289 = case shown="False" w688 {
                          tunnel: w686 -> [w696 w700]
                          tunnel: w681 -> [w695 w699]
                          tunnel: [w697 w698] -> w687
                          frame False {
                            n290 = Add(x=w696, y=w695) -> (x+y=w697:u16)
                          }
                          frame True {
                            n291 = Subtract(x=w700, y=w699) -> (x-y=w698:u16)
                          }
                        }
                      }
                    }
                  }
                }
                n292 = Add(x="BD 1 Frequency 2", y=i64 0 ("f")) -> (x+y=w655:u64)
                "BD1 Frequency Out 2" <- w655
              }
              frame 3 {
                # "Fluorescence period"
              }
            }
            n293 = feedback-in #21(w313) -> ()
            n294 = feedback #21(w313) -> (w312:u16)
            n295 = Select(t=w315, s="Interlace ON/OFF", f="Interlace Off Parameters") -> (s? t:f=w352:u8)
            n296 = Subtract(x=w313, y=w312) -> (x-y=w311:u16)
            n297 = Subtract "The error"(x=w311, y=w310) -> (x-y=w288:u16)
            n298 = case shown="1, Default" w352 {
              tunnel: ["DIO count 1 (ticks)" "DIO count 2 (ticks)" "DIO count 3 (ticks)"] -> w309
              frame 1, Default {
              }
              frame 2 {
              }
              frame 3 {
              }
            }
            n299 = Number To Boolean Array(number=w288) -> (Boolean array=w289:bool[])
            n300 = Or Array Elements(Boolean array=w289) -> (logical OR=w287:bool)
            n301 = Boolean To (0,1)(Boolean=w287) -> (0, 1=w294:i16)
            n302 = To Unsigned Byte Integer(number=w294) -> (unsigned 8bit integer=w291:u8)
            n303 = feedback #22(u8 0) -> (w292:u8)
            n304 = Add(x=w291, y=w292) -> (x+y=w290:u8)
            "DIO Late Counter" <- w290
            n305 = feedback-in #22(w290) -> ()
            n306 = Subtract(x=w309, y=w288) -> (x-y=w308:u16)
            n307 = Split Number(x=w349) -> (hi(x)=w348:u32, lo(x)=w347:u32)
            n308 = Split Number(x=w338) -> (hi(x)=w343:u32, lo(x)=w342:u32)
            n309 = Boolean To (0,1)(Boolean="+ phase (DIO)") -> (0, 1=w305:i16)
            n310 = Split Number(x=w348) -> (lo(x)=w346:u16)  [unwired: 1 out]
            n311 = Split Number(x=w347) -> (hi(x)=w345:u16, lo(x)=w344:u16)
            n312 = Split Number(x=w343) -> (lo(x)=w341:u16)  [unwired: 1 out]
            n313 = Split Number(x=w342) -> (hi(x)=w340:u16, lo(x)=w339:u16)
            n314 = Split Number(x=w298) -> (hi(x)=w300:u8, lo(x)=w299:u8)
            n315 = Split Number(x=w295) -> (hi(x)=w297:u8, lo(x)=w296:u8)
            n316 = Split Number(x=w346) -> (hi(x)=w337:u8, lo(x)=w336:u8)
            n317 = Split Number(x=w345) -> (hi(x)=w335:u8, lo(x)=w334:u8)
            n318 = Split Number(x=w341) -> (hi(x)=w330:u8, lo(x)=w329:u8)
            n319 = Split Number(x=w344) -> (hi(x)=w333:u8, lo(x)=w332:u8)
            n320 = Split Number(x=w340) -> (hi(x)=w328:u8, lo(x)=w327:u8)
            n321 = Split Number(x=w339) -> (hi(x)=w326:u8, lo(x)=w325:u8)
            n322 = Multiply(x=w305, y="Phase count adjustment (DIO)") -> (x*y=w301:i16)
            n323 = feedback #23(i16 0) -> (w303:i16)
            n324 = Subtract(x=w303, y=w301) -> (x-y=w302:i16)
            "DIO Relative phase" <- w302
            n325 = feedback-in #23(w302) -> ()
            n326 = Add(x=w308, y=w301) -> (x+y=w307:u16)
            n327 = Build Array "BD 1 A Stack"(w300, w299) -> (w322:u8[])
            n328 = Build Array "BD 2 A Stack"(w297, w296) -> (w321:u8[])
            n329 = Build Array "BD 1 nu Stack"(w337, w336, w335, w334, w333, w332) -> (w331:u8[])
            n330 = Build Array "BD 2 nu Stack"(w330, w329, w328, w327, w326, w325) -> (w324:u8[])
            n331 = case shown="2" w279 {
              tunnel: [w392 w395] -> w320
              tunnel: [u8 10 u8 4] -> w323
              tunnel: "Swap F1 and F2" -> [w393 w395]
              frame 2 {
                # "F2"
                n332 = Not(x=w393) -> (.not. x?=w392:bool)
              }
              frame 1, Default {
                # "low chooses F1"
                # "F1"
              }
            }
            n333 = case "If FPGA is controlling (toggling) RF synth" shown="True" w319 {
              tunnel: w331 -> [_ w368]
              tunnel: w324 -> [_ w367]
              tunnel: w323 -> [_ w366]
              tunnel: w322 -> [_ w365]
              tunnel: w321 -> [_ w364]
              frame False {
              }
              frame True {
                # "Write next amp.\n(wait until beginning of next loop iteration to update)"
                n334 = flat-sequence "Update the next F1 and F2 frequency value (the actual frequency won't change until FSK is switched).\nThen load the next amplitude value into buffer, but don't update it until the next cycle." {
                  tunnel: w367 -> [w370]
                  tunnel: w368 -> [w371]
                  tunnel: [w371] -> w363
                  tunnel: [w370] -> w362
                  tunnel: w366 -> [w372]
                  tunnel: w363 -> [w374]
                  tunnel: w362 -> [w373]
                  tunnel: w365 -> [w385]
                  tunnel: w364 -> [w384]
                  frame #0 {
                    # "To possibly send\nthese writes to very\nend of loop (for x and\ny phase adjust)"
                    n335 = call "Wait8"("Count(Ticks)"="Next trap write delay (ticks)") -> ()  [unwired: 1 out]
                  }
                  frame #1 {
                    n336 = for {
                      tunnel: w374 -> [w380] mode=indexing
                      tunnel: w373 -> [w379] mode=indexing
                      tunnel: w372 -> [w377]
                      i -> [w378]
                      # "Write next freq."
                      n337 = To Unsigned Byte Integer(number=w378) -> (unsigned 8bit integer=w375:u8)
                      n338 = Add(x=w377, y=w375) -> (x+y=w376:u8)
                      n339 = call "write to RF synth bd.vi"("Address Byte"=w376, "BD 2 Byte"=w379, "BD 1 Byte"=w380) -> ()
                    }
                  }
                  frame #2 {
                    w381 = TRUE ("Connector1/DIO15")
                    # "send udclk high\n(BD 1 and 2)"
                    n340 = xnode "FPGA I/O Node"("Connector1/DIO30"=w381, "Connector1/DIO29"=w381) -> ()  [unwired: 2 in, 2 out]
                  }
                  frame #3 {
                    w382 = FALSE ("Connector1/DIO15")
                    n341 = xnode "FPGA I/O Node"("Connector1/DIO30"=w382, "Connector1/DIO29"=w382) -> ()  [unwired: 2 in, 2 out]
                  }
                  frame #4 {
                    n342 = for {
                      tunnel: w385 -> [w391] mode=indexing
                      tunnel: w384 -> [w390] mode=indexing
                      tunnel: u8 33 -> [w388]
                      i -> [w389]
                      n343 = To Unsigned Byte Integer(number=w389) -> (unsigned 8bit integer=w386:u8)
                      n344 = Add(x=w388, y=w386) -> (x+y=w387:u8)
                      n345 = call "write to RF synth bd.vi"("Address Byte"=w387, "BD 2 Byte"=w390, "BD 1 Byte"=w391) -> ()
                    }
                  }
                }
              }
            }
          }
        }
      }
    }
  }
  n346 = while "APD 1 Counter" {
    tunnel: w4 -> [_]
    stop <- FALSE stop-if-true
    n347 = flat-sequence {
      frame #0 {
        n348 = xnode "FPGA I/O Method Node"("FPGA I/O In"=refnum<k21> "Connector0/DIO0" ("APD 1 DO"), "Timeout"=-1) -> ()  [unwired: 2 out]
      }
      frame #1 {
        n349 = local read "APD1 int gate"() -> (w711:bool)
        n350 = case shown="True" w711 {
          frame False {
          }
          frame True {
            n351 = local read "APD1 out state"() -> (w712:bool)
            n352 = case shown="True" w712 {
              frame False {
                n353 = local read "APD 1 Counts 0"() -> (w714:u32)
                n354 = Increment(x=w714) -> (x+1=→"APD 1 Counts 0":u32)
              }
              frame True {
                n355 = local read "APD 1 Counts 1"() -> (w716:u32)
                n356 = Increment(x=w716) -> (x+1=→"APD 1 Counts 1":u32)
              }
            }
          }
        }
      }
    }
  }
  n357 = disable-structure shown="Disabled" {
    disable-tunnel: u16 0 -> [w718 _]
    disable-tunnel: w4 -> [w717 _]
    frame Disabled {
      n358 = while "Green and red fluorescent laser interlacing (Current AO to IA 532 nm AOM ME amp)." {
        shift-right: [w727] -> _
        shift-left: w717 -> [w730]
        shift-right: [w724] -> _
        shift-left: w718 -> [w722]
        shift-right: [w721] -> _
        shift-left: w718 -> [w720]
        stop <- FALSE stop-if-true
        n359 = flat-sequence {
          tunnel: w730 -> [w734]
          tunnel: [w735] -> w729
          tunnel: [w734] -> w728
          tunnel: [w733] -> w723
          tunnel: w722 -> [w733]
          tunnel: w720 -> [w732]
          tunnel: [w732] -> w719
          tunnel: [w739] -> w726
          tunnel: w729 -> [w739]
          tunnel: [w738] -> w725
          tunnel: w728 -> [w738]
          tunnel: w723 -> [w737]
          tunnel: w719 -> [w736]
          tunnel: [w760] -> w727
          tunnel: [w776] -> w724
          tunnel: w726 -> [w787]
          tunnel: w725 -> [w784]
          tunnel: [w744] -> w721
          frame #0 {
            n360 = call "Loop Timer10"("Count(Ticks)"=w734) -> ("Tick Count(Ticks)"=w735:u16)
          }
          frame #1 {
            n361 = xnode "FPGA I/O Node"("Chassis2/Mod1/AO0"=w737, "Chassis2/Mod1/AO1"=w736) -> ()  [unwired: 2 in, 2 out]
          }
          frame #2 {
            # "Design note:\n\nThese two laser controls are in the same loop\nbecause the expansion current AI cannot separately\ntime the outputs fast enough for us.  Apparently\nit is because of communication time between the\nexpansion card and the fpga.\n\nSo the two analog control signals have the same timing\nand profile, but independent amplitudes to independently\ncontrol the intensity and feedback for each laser."
            n362 = feedback #24(TRUE) -> (w740:bool)
            n363 = Not(x=w740) -> (.not. x?=w741:bool)
            n364 = feedback-in #24(w741) -> ()
            n365 = Subtract(x="Green interlace OFF count 2", y="Green int current ON count adj") -> (x-y=w769:u16)
            n366 = feedback-in #25(w787) -> ()
            n367 = feedback #25(w787) -> (w786:u16)
            n368 = Add(x="Green int current ON count adj", y="Green interlace ON count 2") -> (x+y=w770:u16)
            n369 = Subtract(x=w787, y=w786) -> (x-y=w785:u16)
            n370 = Select(t=w770, s=w741, f=w769) -> (s? t:f=w781:u16)
            n371 = Subtract(x=w785, y=w784) -> (x-y=w753:u16)
            n372 = case shown="2" "RI Operating Mode 2" {
              tunnel: [TRUE FALSE w793] -> w742
              tunnel: w740 -> [_ _ w790]
              frame 0, Default {
              }
              frame 1 {
              }
              frame 2 {
                n373 = Not(x=w790) -> (.not. x?=w792:bool)
                n374 = Select(t=w792, s="Invert RI 2", f=w790) -> (s? t:f=w793:bool)
              }
            }
            n375 = Subtract(x=w781, y=w753) -> (x-y=w764:u16)
            n376 = case shown="0, Default" "Operating Mode 2" {
              tunnel: [TRUE FALSE w827] -> w745
              tunnel: w740 -> [_ _ w824]
              frame 0, Default {
              }
              frame 1 {
              }
              frame 2 {
                n377 = Not(x=w824) -> (.not. x?=w826:bool)
                n378 = Select(t=w826, s="Invert GI 2", f=w824) -> (s? t:f=w827:bool)
              }
            }
            n379 = Number To Boolean Array(number=w753) -> (Boolean array=w754:bool[])
            n380 = Boolean To (0,1)(Boolean="+ phase (GI) 2") -> (0, 1=w766:i16)
            n381 = Or Array Elements(Boolean array=w754) -> (logical OR=w752:bool)
            n382 = Boolean To (0,1)(Boolean=w752) -> (0, 1=w759:i16)
            n383 = Multiply(x=w766, y="Phase count adjustment (GI) 2") -> (x*y=w762:i16)
            n384 = To Unsigned Byte Integer(number=w759) -> (unsigned 8bit integer=w755:u8)
            n385 = Add(x=w764, y=w762) -> (x+y=w760:u16)
            n386 = feedback #26(u8 0) -> (w757:u8)
            n387 = Add(x=w755, y=w757) -> (x+y=w756:u8)
            "GI Late Counter 2" <- w756
            n388 = feedback-in #26(w756) -> ()
            n389 = feedback #27(i16 0) -> (w763:i16)
            n390 = Subtract(x=w763, y=w762) -> (x-y=w761:i16)
            "GI Relative phase 2" <- w761
            n391 = feedback-in #27(w761) -> ()
            n392 = And(x=w745, y="Green FB On/Off") -> (x .and. y?=w771:bool)
            n393 = And(x=w742, y="Red FB On/Off") -> (x .and. y?=w751:bool)
            n394 = case shown="False" w771 {
              tunnel: "Current Out" -> [w808 _]
              tunnel: [w808 w817] -> w775
              frame False {
              }
              frame True {
                n395 = local read "Green FB Sum"() -> (w813:i16)
                n396 = Bundle("P3"="P3", "I3"="I3", "D3"="D3") -> (w809:cluster{"P3":i16, "I3":i16, "D3":i16})  [unwired: 1 in]
                n397 = call "Slower PID.vi"("process variable"=w813, "reset?"="Green FB Reset", "setpoint"="Green FB Setpoint", "PID gains (x 2^8)"=w809, "output range"=cluster{"output high":i16, "output low":i16} {"output high"=32767, "output low"=-32768} ("Green FB output range")) -> ("output"=w820:i16)  [unwired: 10 out]
                n398 = To Long Integer(number=w820) -> (32bit integer=w814:i32)
                n399 = Add(x=w814, y=32768) -> (x+y=w816:i32)
                n400 = To Unsigned Word Integer(number=w816) -> (unsigned 16bit integer=w817:u16)
              }
            }
            n401 = case shown="True" w751 {
              tunnel: "RI Current Out" -> [w794 _]
              tunnel: [w794 w803] -> w747
              frame False {
              }
              frame True {
                n402 = local read "Red FB Intensity"() -> (w799:i16)
                n403 = Bundle("P4"="P4", "I4"="I4", "D4"="D4") -> (w795:cluster{"P4":i16, "I4":i16, "D4":i16})  [unwired: 1 in]
                n404 = call "Slower PID.vi"("process variable"=w799, "reset?"="Red FB Reset", "setpoint"="Red FB Setpoint", "PID gains (x 2^8)"=w795, "output range"=cluster{"output high":i16, "output low":i16} {"output high"=32767, "output low"=-32768} ("Green FB output range")) -> ("output"=w806:i16)  [unwired: 10 out]
                n405 = To Long Integer(number=w806) -> (32bit integer=w800:i32)
                n406 = Add(x=w800, y=32768) -> (x+y=w802:i32)
                n407 = To Unsigned Word Integer(number=w802) -> (unsigned 16bit integer=w803:u16)
              }
            }
            n408 = Boolean To (0,1)(Boolean=w745) -> (0, 1=w777:i16)
            n409 = Boolean To (0,1)(Boolean=w742) -> (0, 1=w746:i16)
            n410 = To Unsigned Word Integer(number=w777) -> (unsigned 16bit integer=w774:u16)
            n411 = To Unsigned Word Integer(number=w746) -> (unsigned 16bit integer=w748:u16)
            n412 = Multiply(x=w774, y=w775) -> (x*y=w776:u16)
            n413 = Multiply(x=w748, y=w747) -> (x*y=w744:u16)
          }
        }
      }
    }
    frame Enabled {
    }
  }
  n414 = while "APD 2 Counter" {
    tunnel: w4 -> [_]
    stop <- FALSE stop-if-true
    n415 = flat-sequence {
      frame #0 {
        n416 = xnode "FPGA I/O Method Node"("FPGA I/O In"=refnum<k21> "Connector0/DIO1" ("APD 2 DO"), "Timeout"=-1) -> ()  [unwired: 2 out]
      }
      frame #1 {
        n417 = local read "APD2 int gate"() -> (w831:bool)
        n418 = case shown="True" w831 {
          frame False {
          }
          frame True {
            n419 = local read "APD2 out state"() -> (w832:bool)
            n420 = case shown="False" w832 {
              frame False {
                n421 = local read "APD 2 Counts 0"() -> (w834:u32)
                n422 = Increment(x=w834) -> (x+1=→"APD 2 Counts 0":u32)
              }
              frame True {
                n423 = local read "APD 2 Counts 1"() -> (w836:u32)
                n424 = Increment(x=w836) -> (x+1=→"APD 2 Counts 1":u32)
              }
            }
          }
        }
      }
    }
  }
  n425 = while "532 nm green fluorescent laser interlacing (DO to IA 532 nm AOM ME amp)." {
    shift-right: [w840] -> _
    shift-left: w4 -> [w845]
    shift-right: [w839] -> _
    shift-left: w5 -> [w837]
    stop <- FALSE stop-if-true
    n426 = flat-sequence {
      tunnel: w845 -> [w848]
      tunnel: [w849] -> w843
      tunnel: [w848] -> w841
      tunnel: [w847] -> w838
      tunnel: w837 -> [w847]
      tunnel: [w852] -> w844
      tunnel: w843 -> [w852]
      tunnel: [w851] -> w842
      tunnel: w841 -> [w851]
      tunnel: w838 -> [w850]
      tunnel: [w861] -> w840
      tunnel: w844 -> [w881]
      tunnel: w842 -> [w878]
      tunnel: [w870] -> w839
      frame #0 {
        n427 = call "Loop Timer4"("Count(Ticks)"=w848) -> ("Tick Count(Ticks)"=w849:u16)
      }
      frame #1 {
        n428 = xnode "FPGA I/O Node"("Connector1/DIO34"=w850, "Connector1/DIO38"=w850, "Connector1/DIO39"=w850) -> ()  [unwired: 3 in, 3 out]
      }
      frame #2 {
        n429 = feedback-in #28(w881) -> ()
        n430 = feedback #28(w881) -> (w880:u16)
        n431 = Subtract(x=w881, y=w880) -> (x-y=w879:u16)
        n432 = Subtract(x=w879, y=w878) -> (x-y=w854:u16)
        n433 = Number To Boolean Array(number=w854) -> (Boolean array=w855:bool[])
        n434 = Or Array Elements(Boolean array=w855) -> (logical OR=w853:bool)
        n435 = Boolean To (0,1)(Boolean="+ phase (GI)") -> (0, 1=w866:i16)
        n436 = Multiply(x=w866, y="Phase count adjustment (GI)") -> (x*y=w863:i16)
        n437 = Boolean To (0,1)(Boolean=w853) -> (0, 1=w860:i16)
        n438 = To Unsigned Byte Integer(number=w860) -> (unsigned 8bit integer=w857:u8)
        n439 = feedback #29(i16 0) -> (w864:i16)
        n440 = feedback #30(u8 0) -> (w858:u8)
        n441 = Add(x=w857, y=w858) -> (x+y=w856:u8)
        "GI Late Counter" <- w856
        n442 = feedback-in #30(w856) -> ()
        n443 = Subtract(x=w864, y=w863) -> (x-y=w862:i16)
        "GI Relative phase" <- w862
        n444 = feedback-in #29(w862) -> ()
        n445 = feedback #31(TRUE) -> (w873:bool)
        n446 = case shown="2" "Operating Mode" {
          tunnel: [TRUE FALSE w887] -> w870
          tunnel: w873 -> [_ _ w884]
          frame 0, Default {
          }
          frame 1 {
          }
          frame 2 {
            n447 = Not(x=w884) -> (.not. x?=w886:bool)
            n448 = Select(t=w886, s="Invert GI", f=w884) -> (s? t:f=w887:bool)
          }
        }
        n449 = Not(x=w873) -> (.not. x?=w869:bool)
        n450 = Select(t="Green interlace ON count", s=w869, f="Green interlace OFF count") -> (s? t:f=w875:u16)
        n451 = Subtract(x=w875, y=w854) -> (x-y=w867:u16)
        n452 = Add(x=w867, y=w863) -> (x+y=w861:u16)
        n453 = feedback-in #31(w869) -> ()
      }
    }
  }
  n454 = while "Excitation laser intensity feedback measurement (all lasers)" {
    shift-right: [w888] -> _
    shift-left: w4 -> [w893]
    stop <- FALSE stop-if-true
    n455 = flat-sequence {
      tunnel: w893 -> [w895]
      tunnel: [w896] -> w891
      tunnel: [w895] -> w889
      tunnel: [w902] -> w892
      tunnel: w891 -> [w902]
      tunnel: [w901] -> w890
      tunnel: w889 -> [w901]
      tunnel: [w914] -> w888
      tunnel: w892 -> [w925]
      tunnel: w890 -> [w922]
      frame #0 {
        n456 = call "Loop Timer9"("Count(Ticks)"=w895) -> ("Tick Count(Ticks)"=w896:u16)
      }
      frame #1 {
        # "Design note:\n\nAll lasers need to be measured at the same \ntime because the AI expansion module\ncannot independently time the measurements\nwithin our requirements: their is dead time.\n\nThis probably wouldn't be an issue with the built\nin AI on the fpga board itself."
        n457 = xnode "FPGA I/O Node"("Connector1/DIO35"=TRUE) -> ("Chassis2/Mod2/AI2"=→"Blue Intensity":i16, "Chassis2/Mod2/AI1"=→"Red FB Intensity":i16, "Chassis2/Mod2/AI0"=→"Green FB Sum":i16)  [unwired: 4 in, 4 out]
      }
      frame #2 {
        n458 = feedback-in #32(w925) -> ()
        n459 = feedback #32(w925) -> (w924:u16)
        n460 = Subtract(x=w925, y=w924) -> (x-y=w923:u16)
        n461 = xnode "FPGA I/O Node"("Connector1/DIO35"=FALSE) -> ()  [unwired: 1 in, 1 out]
        n462 = Subtract(x=w923, y=w922) -> (x-y=w904:u16)
        n463 = Subtract(x="Green FB Count", y=w904) -> (x-y=w918:u16)
        n464 = Number To Boolean Array(number=w904) -> (Boolean array=w905:bool[])
        n465 = Or Array Elements(Boolean array=w905) -> (logical OR=w903:bool)
        n466 = Boolean To (0,1)(Boolean="+ phase (Green FB)") -> (0, 1=w916:i16)
        n467 = Boolean To (0,1)(Boolean=w903) -> (0, 1=w910:i16)
        n468 = Multiply(x=w916, y="Phase count adjustment (Green FB)") -> (x*y=w911:i16)
        n469 = Add(x=w918, y=w911) -> (x+y=w914:u16)
        n470 = To Unsigned Byte Integer(number=w910) -> (unsigned 8bit integer=w907:u8)
        n471 = feedback #33(i16 0) -> (w913:i16)
        n472 = Subtract(x=w913, y=w911) -> (x-y=w912:i16)
        "Green FB Relative Phase" <- w912
        n473 = feedback-in #33(w912) -> ()
        n474 = feedback #34(u8 0) -> (w908:u8)
        n475 = Add(x=w907, y=w908) -> (x+y=w906:u8)
        "Green Late Counter" <- w906
        n476 = feedback-in #34(w906) -> ()
      }
    }
  }
  n477 = while "MCL stage control" {
    shift-right: [w938] -> _
    shift-left: w4 -> [w941]
    shift-right: [w931] -> _
    shift-left: w12 -> [w928]
    shift-right: [w930] -> _
    shift-left: w11 -> [w926]
    stop <- FALSE stop-if-true
    n478 = flat-sequence {
      tunnel: w941 -> [w945]
      tunnel: [w946] -> w937
      tunnel: [w945] -> w935
      tunnel: [w944] -> w929
      tunnel: w928 -> [w944]
      tunnel: [w943] -> w927
      tunnel: w926 -> [w943]
      tunnel: w937 -> [w950]
      tunnel: [w950] -> w936
      tunnel: w935 -> [w949]
      tunnel: [w949] -> w934
      tunnel: w929 -> [w948]
      tunnel: w927 -> [w947]
      tunnel: w936 -> [w958]
      tunnel: w934 -> [w957]
      tunnel: [w958] -> w940
      tunnel: [w957] -> w939
      tunnel: [w956] -> w933
      tunnel: [w955] -> w932
      tunnel: [w1030] -> w938
      tunnel: w940 -> [w1037]
      tunnel: w939 -> [w1034]
      tunnel: w933 -> [w1032]
      tunnel: w932 -> [w1031]
      tunnel: [w1032] -> w931
      tunnel: [w1031] -> w930
      frame #0 {
        n479 = call "Loop Timer5"("Count(Ticks)"=w945) -> ("Tick Count(Ticks)"=w946:u32)
      }
      frame #1 {
        n480 = xnode "FPGA I/O Node"("Connector0/AO1"=w948, "Connector0/AO2"=w947) -> ()  [unwired: 2 in, 2 out]
      }
      frame #2 {
        n481 = local read "Scanning MCL"() -> (w970:bool)
        n482 = Or(x=w970, y="Start scan (MCL)") -> (x .or. y?=w965:bool)
        n483 = Not(x="Abort scan (MCL)") -> (.not. x?=w963:bool)
        n484 = And(x=w963, y=w965) -> (x .and. y?=w962:bool)
        n485 = case "Raster scan" shown="True" w962 {
          tunnel: [w971 w1014] -> w967
          tunnel: "Start scan (MCL)" -> [_ w999]
          tunnel: [w971 w975] -> w951
          frame False {
            w971 = i16 0
            n486 = local write "Scanning MCL"(FALSE ("scanning")) -> ()
          }
          frame True {
            w985 = i16 0
            w984 = u64 0
            # "scan incr."
            # "freq. incr. mult."
            # "count steps"
            # "count number of cycles"
            n487 = feedback #35(w984) -> (w1011:u64)
            n488 = Select(t=w984, s=w999, f=w1011) -> (s? t:f=w1013:u64)
            n489 = Increment(x=w1013) -> (x+1=w1010:u64)
            n490 = Greater?(x="Cycles per step (MCL)", y=w1010) -> (0:w994:bool)
            n491 = Select(t=w1010, s=w994, f=w984) -> (s? t:f=w1009:u64)
            n492 = feedback-in #35(w1009) -> ()
            n493 = feedback #36(w984) -> (w1008:u64)
            n494 = Select(t=w984, s=w999, f=w1008) -> (s? t:f=w1003:u64)
            n495 = Increment(x=w1003) -> (x+1=w1007:u64)
            n496 = Add(x="Scan steps (MCL)", y="Scan steps (MCL)") -> (x+y=w1006:u64)
            n497 = Select(t=w1003, s=w994, f=w1007) -> (s? t:f=w989:u64)
            n498 = Greater?(x=w1006, y=w989) -> (0:w988:bool)
            n499 = Select(t=w989, s=w988, f=w984) -> (s? t:f=w1004:u64)
            n500 = feedback-in #36(w1004) -> ()
            n501 = Equal?(x="Scan steps (MCL)", y=w989) -> (x = y?=w993:bool)
            n502 = Greater?(x="Scan steps (MCL)", y=w1003) -> (0:w1002:bool)
            n503 = feedback #37(w985) -> (w1005:i16)
            n504 = Select(t=w985, s=w999, f=w1005) -> (s? t:f=w991:i16)
            n505 = Increment(x=w991) -> (x+1=w1001:i16)
            n506 = Decrement(x=w991) -> (x-1=w1000:i16)
            n507 = Select(t=w1001, s=w1002, f=w1000) -> (s? t:f=w992:i16)
            n508 = Select(t=w991, s=w993, f=w992) -> (s? t:f=w990:i16)
            n509 = Select(t=w991, s=w994, f=w990) -> (s? t:f=w986:i16)
            n510 = Select(t=w986, s=w988, f=w985) -> (s? t:f=w987:i16)
            n511 = feedback-in #37(w987) -> ()
            n512 = feedback #38(w984) -> (w998:u64)
            n513 = Select(t=w984, s=w999, f=w998) -> (s? t:f=w973:u64)
            n514 = Increment(x=w973) -> (x+1=w995:u64)
            n515 = Select(t=w973, s=w988, f=w995) -> (s? t:f=w974:u64)
            n516 = Greater?(x="Number of scans (MCL)", y=w974) -> (0:w981:bool)
            n517 = Multiply(x="Scan freq.  increment (MCL)", y=w991) -> (x*y=w1014:i16)
            n518 = Select(t=TRUE, s="Cont. Scan (MCL)", f=w981) -> (s? t:f=w980:bool)
            "Scanning MCL" <- w980
            n519 = Select(t=w974, s=w980, f=w984) -> (s? t:f=w996:u64)
            n520 = feedback-in #38(w996) -> ()
            n521 = Increment(x=w974) -> (x+1=→"Scan I (MCL)":u64)
            n522 = To Word Integer(number=w973) -> (16bit integer=w976:i16)
            n523 = Multiply(x=w976, y="Scan freq.  increment (MCL)") -> (x*y=w975:i16)
          }
        }
        n524 = Select(t=w951, s="1D or 2D Scan?", f=i16 0) -> (s? t:f=w952:i16)
        n525 = Select(t=w952, s="MCL Scan Axis", f=w967) -> (s? t:f=w966:i16)
        n526 = Select(t=w967, s="MCL Scan Axis", f=w952) -> (s? t:f=w968:i16)
        n527 = Add(x=w966, y="AO2") -> (x+y=w955:i16)
        n528 = Add(x="AO1", y=w968) -> (x+y=w956:i16)
      }
      frame #3 {
        n529 = feedback-in #39(w1037) -> ()
        n530 = feedback #39(w1037) -> (w1036:u32)
        n531 = Boolean To (0,1)(Boolean="+ phase (MCL)") -> (0, 1=w1028:i16)
        n532 = Subtract(x=w1037, y=w1036) -> (x-y=w1035:u32)
        n533 = Multiply(x=w1028, y="Phase count adjustment (MCL)") -> (x*y=w1024:i16)
        n534 = Subtract(x=w1035, y=w1034) -> (x-y=w1016:u32)
        n535 = Subtract(x="MCL count", y=w1016) -> (x-y=w1026:u32)
        n536 = feedback #40(i16 0) -> (w1025:i16)
        n537 = Subtract(x=w1025, y=w1024) -> (x-y=w1023:i16)
        "MCL Relative Phase" <- w1023
        n538 = feedback-in #40(w1023) -> ()
        n539 = Number To Boolean Array(number=w1016) -> (Boolean array=w1017:bool[])
        n540 = Or Array Elements(Boolean array=w1017) -> (logical OR=w1015:bool)
        n541 = Boolean To (0,1)(Boolean=w1015) -> (0, 1=w1022:i16)
        n542 = Add(x=w1026, y=w1024) -> (x+y=w1030:u32)
        n543 = To Unsigned Byte Integer(number=w1022) -> (unsigned 8bit integer=w1019:u8)
        n544 = feedback #41(u8 0) -> (w1020:u8)
        n545 = Add(x=w1019, y=w1020) -> (x+y=w1018:u8)
        "MCL Late Counter" <- w1018
        n546 = feedback-in #41(w1018) -> ()
      }
    }
  }
  n547 = while "Control APD data integration - stream to host" {
    shift-right: [w1042] -> _
    shift-left: w8 -> [w1047]
    stop <- FALSE stop-if-true
    n548 = flat-sequence {
      tunnel: w1047 -> [w1049]
      tunnel: [w1050] -> w1045
      tunnel: [w1049] -> w1043
      tunnel: [w1060] -> w1046
      tunnel: w1045 -> [w1060]
      tunnel: [w1059] -> w1044
      tunnel: w1043 -> [w1059]
      tunnel: [w1058] -> w1041
      tunnel: [w1057] -> w1040
      tunnel: [w1051] -> w1039
      tunnel: [w1102] -> w1042
      tunnel: w1046 -> [w1112]
      tunnel: w1044 -> [w1109]
      tunnel: w1041 -> [w1095]
      tunnel: w1040 -> [w1094]
      tunnel: w1039 -> [w1082]
      frame #0 {
        n549 = call "Loop Timer6"("Count(Ticks)"=w1049) -> ("Tick Count(Ticks)"=w1050:u32)
      }
      frame #1 {
        n550 = flat-sequence {
          tunnel: [w1062] -> w1056
          tunnel: w1056 -> [w1065]
          tunnel: [w1069] -> w1055
          tunnel: [w1068] -> w1054
          tunnel: [w1065] -> w1053
          tunnel: [w1064] -> w1052
          tunnel: [w1076] -> w1057
          tunnel: [w1077] -> w1058
          tunnel: w1055 -> [w1077]
          tunnel: w1054 -> [w1076]
          tunnel: w1053 -> [w1075]
          tunnel: w1052 -> [w1074]
          tunnel: [w1074] -> w1051
          frame #0 {
            # "use separate variable so each APD won't\nhave to wait to read"
            n551 = feedback #42(FALSE) -> (w1061:bool)
            "APD1 out state" <- w1061
            "APD2 out state" <- w1061
            "APD3 out state" <- w1061
            n552 = Not(x=w1061) -> (.not. x?=w1062:bool)
            n553 = feedback-in #42(w1062) -> ()
          }
          frame #1 {
            n554 = local read "APD 3 Counts 1"() -> (w1067:u32)
            n555 = local read "APD 3 Counts 0"() -> (w1066:u32)
            n556 = local read "APD 1 Counts 1"() -> (w1073:u32)
            n557 = local read "APD 1 Counts 0"() -> (w1072:u32)
            n558 = local read "APD 2 Counts 1"() -> (w1071:u32)
            n559 = local read "APD 2 Counts 0"() -> (w1070:u32)
            n560 = Select(t=w1067, s=w1065, f=w1066) -> (s? t:f=w1064:u32)
            n561 = Select(t=w1073, s=w1065, f=w1072) -> (s? t:f=w1069:u32)
            n562 = Select(t=w1071, s=w1065, f=w1070) -> (s? t:f=w1068:u32)
          }
          frame #2 {
            n563 = case shown="False" w1075 {
              frame False {
                w1078 = u32 0 ("APD 1 Counts 0")
                n564 = local write "APD 1 Counts 0"(w1078) -> ()
                n565 = local write "APD 2 Counts 0"(w1078) -> ()
                n566 = local write "APD 3 Counts 0"(w1078) -> ()
              }
              frame True {
                w1079 = u32 0 ("APD 1 Counts 1")
                n567 = local write "APD 1 Counts 1"(w1079) -> ()
                n568 = local write "APD 2 Counts 1"(w1079) -> ()
                n569 = local write "APD 3 Counts 1"(w1079) -> ()
              }
            }
          }
        }
      }
      frame #2 {
        n570 = feedback-in #43(w1112) -> ()
        n571 = feedback #43(w1112) -> (w1111:u32)
        n572 = Subtract(x=w1112, y=w1111) -> (x-y=w1110:u32)
        n573 = Subtract(x=w1110, y=w1109) -> (x-y=w1087:u32)
        n574 = case shown="True" "APD to FIFO" {
          tunnel: w1095 -> [_ w1117]
          tunnel: w1094 -> [_ w1115]
          tunnel: w1082 -> [_ w1113]
          frame False {
          }
          frame True {
            n575 = flat-sequence {
              tunnel: 0 ("Timeout") -> [w1119]
              tunnel: w1117 -> [w1120]
              tunnel: [w1119] -> w1116
              tunnel: w1116 -> [w1121]
              tunnel: w1115 -> [w1122]
              tunnel: [w1121] -> w1114
              tunnel: w1114 -> [w1124]
              tunnel: w1113 -> [w1123]
              frame #0 {
                n576 = xnode ("FIFO Write")("Element"=w1120, "Timeout"=w1119) -> ()  [unwired: 1 in, 2 out]
              }
              frame #1 {
                n577 = xnode ("FIFO Write")("Element"=w1122, "Timeout"=w1121) -> ()  [unwired: 1 in, 2 out]
              }
              frame #2 {
                n578 = xnode ("FIFO Write")("Element"=w1123, "Timeout"=w1124) -> ()  [unwired: 1 in, 2 out]
              }
            }
          }
        }
        n579 = Subtract(x="APD Acq Rate Count", y=w1087) -> (x-y=w1103:u32)
        n580 = Number To Boolean Array(number=w1087) -> (Boolean array=w1088:bool[])
        n581 = Or Array Elements(Boolean array=w1088) -> (logical OR=w1086:bool)
        n582 = Boolean To (0,1)(Boolean=w1086) -> (0, 1=w1093:i16)
        n583 = To Unsigned Byte Integer(number=w1093) -> (unsigned 8bit integer=w1090:u8)
        n584 = feedback #44(u8 0) -> (w1091:u8)
        n585 = Add(x=w1090, y=w1091) -> (x+y=w1089:u8)
        "APD Acq Late Counter" <- w1089
        n586 = feedback-in #44(w1089) -> ()
        n587 = Boolean To (0,1)(Boolean="+ phase (APD Acq)") -> (0, 1=w1099:i16)
        n588 = Multiply(x=w1099, y="Phase Count Adjustment (APD Acq)") -> (x*y=w1096:i16)
        n589 = Add(x=w1103, y=w1096) -> (x+y=w1102:u32)
        n590 = feedback #45(i16 0) -> (w1101:i16)
        n591 = Subtract(x=w1101, y=w1096) -> (x-y=w1098:i16)
        "APD Acq Relative Phase" <- w1098
        n592 = feedback-in #45(w1098) -> ()
        n593 = To Word Integer(number=w1095) -> (16bit integer=w1104:i16)
        n594 = To Word Integer(number=w1082) -> (16bit integer=w1083:i16)
        n595 = To Word Integer(number=w1094) -> (16bit integer=w1105:i16)
        n596 = Multiply(x="APD AO scale factor", y=w1105) -> (x*y=w1084:i16)
        n597 = Multiply(x="APD AO scale factor", y=w1083) -> (x*y=w1080:i16)
        n598 = Multiply(x="APD AO scale factor", y=w1104) -> (x*y=w1085:i16)
        n599 = xnode "FPGA I/O Node"("Connector0/AO6"=w1085, "Connector0/AO7"=w1084, "Connector0/AO5"=w1080) -> ()  [unwired: 3 in, 3 out]
      }
    }
  }
  n600 = while "DAQ AI set 1" {
    shift-right: [w1125] -> _
    shift-left: w4 -> [w1130]
    stop <- FALSE stop-if-true
    n601 = flat-sequence {
      tunnel: w1130 -> [w1140]
      tunnel: [w1141] -> w1128
      tunnel: [w1140] -> w1127
      tunnel: [w1151] -> w1138
      tunnel: [w1150] -> w1137
      tunnel: [w1149] -> w1136
      tunnel: [w1148] -> w1135
      tunnel: [w1147] -> w1134
      tunnel: [w1146] -> w1133
      tunnel: [w1145] -> w1132
      tunnel: [w1144] -> w1131
      tunnel: [w1143] -> w1129
      tunnel: w1128 -> [w1143]
      tunnel: w1127 -> [w1142]
      tunnel: [w1142] -> w1126
      tunnel: [w1181] -> w1125
      tunnel: w1138 -> [w1207]
      tunnel: w1137 -> [w1173]
      tunnel: w1136 -> [w1174]
      tunnel: w1135 -> [w1153]
      tunnel: w1134 -> [w1197]
      tunnel: w1133 -> [w1196]
      tunnel: w1132 -> [w1195]
      tunnel: w1131 -> [w1194]
      tunnel: w1129 -> [w1191]
      tunnel: w1126 -> [w1188]
      frame #0 {
        n602 = call "Loop Timer3"("Count(Ticks)"=w1140) -> ("Tick Count(Ticks)"=w1141:u16)
      }
      frame #1 {
        n603 = xnode "FPGA I/O Node"("Connector1/DIO31"=TRUE ("Connector1/DIO33")) -> ("Connector0/AI0"=w1151:i16, "Connector0/AI1"=w1150:i16, "Connector0/AI2"=w1149:i16, "Connector0/AI3"=w1148:i16, "Connector0/AI4"=w1147:i16, "Connector0/AI5"=w1146:i16, "Connector0/AI6"=w1145:i16, "Connector0/AI7"=w1144:i16)  [unwired: 9 in, 9 out]
      }
      frame #2 {
        w1177 = FALSE ("AI to FIFO")
        # "Adjust phase after data acquired if button pressed"
        n604 = feedback #46(i16 1) -> (w1200:i16)
        n605 = Increment(x=w1200) -> (x+1=w1206:i16)
        n606 = Scale By Power Of 2(n="AI1 X Scale", x=w1173) -> (x*2^n=w1171:i16)
        n607 = Greater?(x=w1206, y="N of AI1 Int Acq Sets") -> (0:w1203:bool)
        n608 = Select(t=i16 1, s=w1203, f=w1206) -> (s? t:f=w1205:i16)
        n609 = feedback-in #46(w1205) -> ()
        n610 = Divide(x=w1171, y=w1153) -> (x/y=w1170:fxp<+/-,16,1>)
        n611 = feedback #47(w1177) -> (w1175:bool)
        n612 = feedback #48(w1177) -> (w1193:bool)
        n613 = case shown="2" w1200 {
          tunnel: w1174 -> [w1230 w1237 _]
          tunnel: ["Set 1" "Set 2" "Set 3"] -> w1198
          tunnel: ["AI to FIFO" w1239 w1244] -> w1192
          tunnel: w1193 -> [_ w1239 w1244]
          tunnel: ["Trap Pos to FIFO" w1238 w1243] -> w1176
          tunnel: w1175 -> [_ w1238 w1243]
          tunnel: w1170 -> [w1229 w1236 _]
          tunnel: [w1228 w1234 FALSE] -> w1157
          tunnel: [w1227 w1235 u64 0 ("BD1 Frequency Out 2")] -> w1156
          frame 1, Default {
            n614 = local read "BD1 Frequency Out 1"() -> (w1227:u64)
            n615 = Compound Arithmetic op=AND("Trap Pos to FIFO", "Set 1", "AI to FIFO") -> (w1228:bool)
            "AI2 Y Sum Set 1" <- w1230
            "AI1 X Set 1" <- w1229
          }
          frame 2 {
            n616 = local read "BD1 Frequency Out 2"() -> (w1235:u64)
            n617 = Compound Arithmetic op=AND(w1238, "Set 2", w1239) -> (w1234:bool)
            "AI2 Y Sum Set 2" <- w1237
            "AI1 X Set 2" <- w1236
          }
          frame 3 {
          }
        }
        n618 = And(x=w1198, y=w1192) -> (x .and. y?=w1199:bool)
        n619 = case shown="True" w1199 {
          tunnel: w1207 -> [_ w1258]
          tunnel: w1173 -> [_ w1257]
          tunnel: w1174 -> [_ w1256]
          tunnel: w1153 -> [_ w1255]
          tunnel: w1197 -> [_ w1254]
          tunnel: w1196 -> [_ w1253]
          tunnel: w1195 -> [_ w1252]
          tunnel: w1194 -> [_ w1251]
          tunnel: 0 ("DMA buffer timeout") -> [_ w1260]
          frame False {
          }
          frame True {
            n620 = Build Array(w1258, w1257, w1256, w1255, w1254, w1253, w1252, w1251) -> (w1259:i16[])
            n621 = for {
              tunnel: w1259 -> [w1262] mode=indexing
              tunnel: w1260 -> [w1263]
              tunnel: [w1261] -> w1249 mode=indexing
              n622 = xnode ("FIFO Write")("Element"=w1262, "Timeout"=w1263) -> ("Timed Out?"=w1261:bool)  [unwired: 1 in, 1 out]
            }
            n623 = Or Array Elements(Boolean array=w1249) -> (logical OR=w1246:bool)
            n624 = Boolean To (0,1)(Boolean=w1246) -> (0, 1=w1248:i16)
            n625 = feedback #49(u16 0) -> (w1247:u16)
            n626 = Add(x=w1248, y=w1247) -> (x+y=w1245:u16)
            "Trap AI FIFO Timeout" <- w1245
            n627 = feedback-in #49(w1245) -> ()
          }
        }
        n628 = feedback-in #47(w1176) -> ()
        n629 = feedback-in #48(w1192) -> ()
        n630 = case shown="True" w1157 {
          tunnel: w1156 -> [_ w1213]
          tunnel: [u8 0 w1210] -> w1155
          frame False {
          }
          frame True {
            n631 = Split Number(x=w1213) -> (hi(x)=w1214:u32, lo(x)=w1215:u32)
            n632 = Split Number(x=w1214) -> (lo(x)=w1216:u16)  [unwired: 1 out]
            n633 = Split Number(x=w1215) -> (hi(x)=w1217:u16, lo(x)=w1218:u16)
            n634 = Build Array "BD 1 nu Stack"(w1216, w1217, w1218) -> (w1212:u16[])
            n635 = for {
              tunnel: w1212 -> [w1225] mode=indexing
              shift-right: [w1221] -> w1210
              shift-left: u8 0 -> [w1222]
              n636 = xnode ("FIFO Method Node")("Element"=w1225, "Timeout"="Trap FIFO Set Timeout") -> ("Timed Out?"=w1224:bool)  [unwired: 1 in, 1 out]
              n637 = Boolean To (0,1)(Boolean=w1224) -> (0, 1=w1223:i16)
              n638 = To Unsigned Byte Integer(number=w1223) -> (unsigned 8bit integer=w1220:u8)
              n639 = Add(x=w1220, y=w1222) -> (x+y=w1221:u8)
            }
          }
        }
        n640 = To Unsigned Word Integer(number=w1155) -> (unsigned 16bit integer=w1154:u16)
        n641 = feedback #50(u16 0) -> (w1168:u16)
        n642 = Add(x=w1154, y=w1168) -> (x+y=w1167:u16)
        "Trap Pos FIFO Timeout" <- w1167
        n643 = feedback-in #50(w1167) -> ()
        n644 = feedback-in #51(w1191) -> ()
        n645 = feedback #51(w1191) -> (w1190:u16)
        n646 = Subtract(x=w1191, y=w1190) -> (x-y=w1189:u16)
        n647 = xnode "FPGA I/O Node"("Connector1/DIO31"=FALSE ("Connector1/DIO34")) -> ()  [unwired: 1 in, 1 out]
        n648 = Subtract(x=w1189, y=w1188) -> (x-y=w1159:u16)
        n649 = Boolean To (0,1)(Boolean="+ phase") -> (0, 1=w1184:i16)
        n650 = Multiply(x=w1184, y="Phase count adjustment") -> (x*y=w1178:i16)
        n651 = Subtract(x="ai count", y=w1159) -> (x-y=w1182:u16)
        n652 = Number To Boolean Array(number=w1159) -> (Boolean array=w1160:bool[])
        n653 = feedback #52(i16 0) -> (w1180:i16)
        n654 = Add(x=w1182, y=w1178) -> (x+y=w1181:u16)
        n655 = Subtract(x=w1180, y=w1178) -> (x-y=w1179:i16)
        "Relative phase" <- w1179
        n656 = feedback-in #52(w1179) -> ()
        n657 = Or Array Elements(Boolean array=w1160) -> (logical OR=w1158:bool)
        n658 = Boolean To (0,1)(Boolean=w1158) -> (0, 1=w1165:i16)
        n659 = To Unsigned Byte Integer(number=w1165) -> (unsigned 8bit integer=w1162:u8)
        n660 = feedback #53(u8 0) -> (w1163:u8)
        n661 = Add(x=w1162, y=w1163) -> (x+y=w1161:u8)
        "AI Late Counter" <- w1161
        n662 = feedback-in #53(w1161) -> ()
      }
    }
  }
  n663 = node-c288(w9) -> ()
  n664 = while "APD 3 Counter" {
    tunnel: w4 -> [_]
    stop <- FALSE stop-if-true
    n665 = flat-sequence {
      frame #0 {
        n666 = xnode "FPGA I/O Method Node"("FPGA I/O In"=refnum<k21> "Connector0/DIO2" ("APD 2 DO"), "Timeout"=-1) -> ()  [unwired: 2 out]
      }
      frame #1 {
        n667 = local read "APD3 int gate"() -> (w1267:bool)
        n668 = case shown="True" w1267 {
          frame False {
          }
          frame True {
            n669 = local read "APD3 out state"() -> (w1268:bool)
            n670 = case shown="True" w1268 {
              frame False {
                n671 = local read "APD 3 Counts 0"() -> (w1270:u32)
                n672 = Increment(x=w1270) -> (x+1=→"APD 3 Counts 0":u32)
              }
              frame True {
                n673 = local read "APD 3 Counts 1"() -> (w1272:u32)
                n674 = Increment(x=w1272) -> (x+1=→"APD 3 Counts 1":u32)
              }
            }
          }
        }
      }
    }
  }
  n675 = while "APD 3 Gating" {
    shift-right: [w1276] -> _
    shift-left: w4 -> [w1281]
    shift-right: [w1275] -> _
    shift-left: w7 -> [w1273]
    stop <- FALSE stop-if-true
    n676 = flat-sequence {
      tunnel: w1281 -> [w1284]
      tunnel: [w1285] -> w1279
      tunnel: [w1284] -> w1277
      tunnel: [w1283] -> w1274
      tunnel: w1273 -> [w1283]
      tunnel: [w1288] -> w1280
      tunnel: w1279 -> [w1288]
      tunnel: [w1287] -> w1278
      tunnel: w1277 -> [w1287]
      tunnel: w1274 -> [w1286]
      tunnel: [w1309] -> w1276
      tunnel: w1280 -> [w1320]
      tunnel: w1278 -> [w1317]
      tunnel: [w1289] -> w1275
      frame #0 {
        n677 = call "Loop Timer15"("Count(Ticks)"=w1284) -> ("Tick Count(Ticks)"=w1285:u16)
      }
      frame #1 {
        # "Signal maybe then sent through \na transistor before APD"
        n678 = xnode "FPGA I/O Node"("Connector0/DIO12"=w1286, "Connector0/DIO13"=w1286, "Connector0/DIO14"=w1286, "Connector0/DIO15"=w1286) -> ()  [unwired: 4 in, 4 out]
        "APD3 int gate" <- w1286
      }
      frame #2 {
        n679 = local read "APD Gate OFF Count"() -> (w1294:u16)
        n680 = local read "APD Gate ON Count"() -> (w1295:u16)
        n681 = feedback #54(TRUE) -> (w1314:bool)
        n682 = feedback-in #55(w1320) -> ()
        n683 = feedback #55(w1320) -> (w1319:u16)
        n684 = Not(x=w1314) -> (.not. x?=w1312:bool)
        n685 = feedback-in #54(w1312) -> ()
        n686 = Subtract(x=w1320, y=w1319) -> (x-y=w1318:u16)
        n687 = Select(t=w1295, s=w1312, f=w1294) -> (s? t:f=w1316:u16)
        n688 = Subtract(x=w1318, y=w1317) -> (x-y=w1297:u16)
        n689 = Subtract(x=w1316, y=w1297) -> (x-y=w1308:u16)
        n690 = Number To Boolean Array(number=w1297) -> (Boolean array=w1298:bool[])
        n691 = Or Array Elements(Boolean array=w1298) -> (logical OR=w1296:bool)
        n692 = Boolean To (0,1)(Boolean=w1296) -> (0, 1=w1303:i16)
        n693 = Boolean To (0,1)(Boolean="+ phase (APD 3 Gate)") -> (0, 1=w1306:i16)
        n694 = To Unsigned Byte Integer(number=w1303) -> (unsigned 8bit integer=w1300:u8)
        n695 = Multiply(x=w1306, y="Phase count adjustment (APD 3 Gate)") -> (x*y=w1304:i16)
        n696 = feedback #56(u8 0) -> (w1301:u8)
        n697 = Add(x=w1300, y=w1301) -> (x+y=w1299:u8)
        "APD 3 Gate Late Counter" <- w1299
        n698 = feedback-in #56(w1299) -> ()
        n699 = Add(x=w1308, y=w1304) -> (x+y=w1309:u16)
        n700 = feedback #57(i16 0) -> (w1311:i16)
        n701 = Subtract(x=w1311, y=w1304) -> (x-y=w1310:i16)
        "APD 3 Gate Relative Phase" <- w1310
        n702 = feedback-in #57(w1310) -> ()
        n703 = local read "APD Gate Operating Mode"() -> (w1293:u8)
        n704 = case shown="2" w1293 {
          tunnel: [TRUE FALSE w1323] -> w1290
          tunnel: w1314 -> [_ _ w1323]
          frame 0, Default {
          }
          frame 1 {
          }
          frame 2 {
          }
        }
        n705 = local read "Invert APD Gate"() -> (w1292:bool)
        n706 = Not(x=w1290) -> (.not. x?=w1291:bool)
        n707 = Select(t=w1291, s=w1292, f=w1290) -> (s? t:f=w1289:bool)
      }
    }
  }
  n708 = disable-structure shown="Disabled" {
    disable-tunnel: w5 -> [w1325 _]
    disable-tunnel: w4 -> [w1324 _]
    frame Disabled {
      n709 = while "633 nm red  fluorescent laser interlacing (DO to IA 633 nm AOM ME amp)." {
        shift-right: [w1329] -> _
        shift-left: w1324 -> [w1334]
        shift-right: [w1328] -> _
        shift-left: w1325 -> [w1326]
        stop <- FALSE stop-if-true
        n710 = flat-sequence {
          tunnel: w1334 -> [w1337]
          tunnel: [w1338] -> w1332
          tunnel: [w1337] -> w1330
          tunnel: [w1336] -> w1327
          tunnel: w1326 -> [w1336]
          tunnel: [w1341] -> w1333
          tunnel: w1332 -> [w1341]
          tunnel: [w1340] -> w1331
          tunnel: w1330 -> [w1340]
          tunnel: w1327 -> [w1339]
          tunnel: [w1350] -> w1329
          tunnel: w1333 -> [w1370]
          tunnel: w1331 -> [w1367]
          tunnel: [w1359] -> w1328
          frame #0 {
            n711 = call "Loop Timer11"("Count(Ticks)"=w1337) -> ("Tick Count(Ticks)"=w1338:u16)
          }
          frame #1 {
            # "Then to PRL 440 amp"
            n712 = xnode "FPGA I/O Node"("Connector1/DIO32"=w1339) -> ()  [unwired: 1 in, 1 out]
          }
          frame #2 {
            n713 = feedback-in #58(w1370) -> ()
            n714 = feedback #58(w1370) -> (w1369:u16)
            n715 = Subtract(x=w1370, y=w1369) -> (x-y=w1368:u16)
            n716 = Subtract(x=w1368, y=w1367) -> (x-y=w1343:u16)
            n717 = Number To Boolean Array(number=w1343) -> (Boolean array=w1344:bool[])
            n718 = Or Array Elements(Boolean array=w1344) -> (logical OR=w1342:bool)
            n719 = Boolean To (0,1)(Boolean="+ phase (RI)") -> (0, 1=w1355:i16)
            n720 = Multiply(x=w1355, y="Phase count adjustment (RI)") -> (x*y=w1352:i16)
            n721 = Boolean To (0,1)(Boolean=w1342) -> (0, 1=w1349:i16)
            n722 = To Unsigned Byte Integer(number=w1349) -> (unsigned 8bit integer=w1346:u8)
            n723 = feedback #59(i16 0) -> (w1353:i16)
            n724 = feedback #60(u8 0) -> (w1347:u8)
            n725 = Add(x=w1346, y=w1347) -> (x+y=w1345:u8)
            "RI Late Counter" <- w1345
            n726 = feedback-in #60(w1345) -> ()
            n727 = Subtract(x=w1353, y=w1352) -> (x-y=w1351:i16)
            "RI Relative phase" <- w1351
            n728 = feedback-in #59(w1351) -> ()
            n729 = feedback #61(TRUE) -> (w1362:bool)
            n730 = case shown="2" "Red Laser Operating Mode" {
              tunnel: [TRUE FALSE w1376] -> w1359
              tunnel: w1362 -> [_ _ w1373]
              frame 0, Default {
              }
              frame 1 {
              }
              frame 2 {
                n731 = Not(x=w1373) -> (.not. x?=w1375:bool)
                n732 = Select(t=w1375, s="Invert RI", f=w1373) -> (s? t:f=w1376:bool)
              }
            }
            n733 = Not(x=w1362) -> (.not. x?=w1358:bool)
            n734 = Select(t="Red interlace ON count", s=w1358, f="Red interlace OFF count") -> (s? t:f=w1364:u16)
            n735 = Subtract(x=w1364, y=w1343) -> (x-y=w1356:u16)
            n736 = Add(x=w1356, y=w1352) -> (x+y=w1350:u16)
            n737 = feedback-in #61(w1358) -> ()
          }
        }
      }
    }
    frame Enabled {
    }
  }
  n738 = disable-structure shown="Disabled" {
    disable-tunnel: w4 -> [w1377 _]
    frame Disabled {
      n739 = while "Blue fluorescent laser interlacing (AO control direct to laser)." {
        shift-right: [w1384] -> _
        shift-left: w1377 -> [w1387]
        shift-right: [w1381] -> _
        shift-left: i16 0 -> [w1379]
        stop <- FALSE stop-if-true
        n740 = flat-sequence {
          tunnel: w1387 -> [w1390]
          tunnel: [w1391] -> w1386
          tunnel: [w1390] -> w1385
          tunnel: [w1389] -> w1380
          tunnel: w1379 -> [w1389]
          tunnel: [w1394] -> w1383
          tunnel: w1386 -> [w1394]
          tunnel: [w1393] -> w1382
          tunnel: w1385 -> [w1393]
          tunnel: w1380 -> [w1392]
          tunnel: [w1404] -> w1384
          tunnel: [w1420] -> w1381
          tunnel: w1383 -> [w1432]
          tunnel: w1382 -> [w1429]
          frame #0 {
            n741 = call "Loop Timer13"("Count(Ticks)"=w1390) -> ("Tick Count(Ticks)"=w1391:u16)
          }
          frame #1 {
            n742 = xnode "FPGA I/O Node"("Connector0/AO3"=w1392) -> ()  [unwired: 1 in, 1 out]
          }
          frame #2 {
            n743 = Subtract(x="Blue OFF count (AO)", y="Blue current ON count adj (AO)") -> (x-y=w1413:u16)
            n744 = feedback-in #62(w1432) -> ()
            n745 = feedback #62(w1432) -> (w1431:u16)
            n746 = Add(x="Blue current ON count adj (AO)", y="Blue ON count (AO)") -> (x+y=w1414:u16)
            n747 = Subtract(x=w1432, y=w1431) -> (x-y=w1430:u16)
            n748 = Subtract(x=w1430, y=w1429) -> (x-y=w1397:u16)
            n749 = Number To Boolean Array(number=w1397) -> (Boolean array=w1398:bool[])
            n750 = Boolean To (0,1)(Boolean="+ phase (BI AO)") -> (0, 1=w1410:i16)
            n751 = Or Array Elements(Boolean array=w1398) -> (logical OR=w1396:bool)
            n752 = Boolean To (0,1)(Boolean=w1396) -> (0, 1=w1403:i16)
            n753 = Multiply(x=w1410, y="Phase count adjustment (BI AO)") -> (x*y=w1406:i16)
            n754 = To Unsigned Byte Integer(number=w1403) -> (unsigned 8bit integer=w1399:u8)
            n755 = feedback #63(u8 0) -> (w1401:u8)
            n756 = Add(x=w1399, y=w1401) -> (x+y=w1400:u8)
            "BI Late Counter (AO)" <- w1400
            n757 = feedback-in #63(w1400) -> ()
            n758 = feedback #64(i16 0) -> (w1407:i16)
            n759 = Subtract(x=w1407, y=w1406) -> (x-y=w1405:i16)
            "BI Relative phase (AO)" <- w1405
            n760 = feedback-in #64(w1405) -> ()
            n761 = feedback #65(TRUE) -> (w1424:bool)
            n762 = case shown="2" "BI Operating Mode (AO)" {
              tunnel: [TRUE FALSE w1448] -> w1415
              tunnel: w1424 -> [_ _ w1445]
              frame 0, Default {
              }
              frame 1 {
              }
              frame 2 {
                n763 = Not(x=w1445) -> (.not. x?=w1447:bool)
                n764 = Select(t=w1447, s="Invert BI (AO)", f=w1445) -> (s? t:f=w1448:bool)
              }
            }
            n765 = And(x=w1415, y="Blue FB On/Off") -> (x .and. y?=w1416:bool)
            n766 = case shown="True" w1416 {
              tunnel: "BI Current Out" -> [w1433 _]
              tunnel: [w1433 w1435] -> w1419
              frame False {
              }
              frame True {
                n767 = local read "Blue Intensity"() -> (w1434:i16)
                n768 = Bundle("P5"="P5", "I5"="I5", "D5"="D5") -> (w1436:cluster{"P5":i16, "I5":i16, "D5":i16})  [unwired: 1 in]
                n769 = call "Slower PID.vi"("process variable"=w1434, "reset?"="Blue FB Reset", "setpoint"="Blue FB Setpoint", "PID gains (x 2^8)"=w1436, "output range"=cluster{"output high":i16, "output low":i16} {"output high"=32767, "output low"=0} ("Green FB output range")) -> ("output"=w1435:i16)  [unwired: 10 out]
              }
            }
            n770 = Not(x=w1424) -> (.not. x?=w1421:bool)
            n771 = Select(t=w1414, s=w1421, f=w1413) -> (s? t:f=w1426:u16)
            n772 = Subtract(x=w1426, y=w1397) -> (x-y=w1408:u16)
            n773 = Add(x=w1408, y=w1406) -> (x+y=w1404:u16)
            n774 = feedback-in #65(w1421) -> ()
            n775 = Boolean To (0,1)(Boolean=w1415) -> (0, 1=w1395:i16)
            n776 = Multiply(x=w1395, y=w1419) -> (x*y=w1420:i16)
          }
        }
      }
    }
    frame Enabled {
    }
  }
  n777 = disable-structure shown="Disabled" {
    disable-tunnel: w5 -> [w1450 _]
    disable-tunnel: w4 -> [w1449 _]
    frame Disabled {
      n778 = while "473 nm blue  fluorescent laser interlacing (DO to blue laser digital control input)." {
        shift-right: [w1454] -> _
        shift-left: w1449 -> [w1459]
        shift-right: [w1453] -> _
        shift-left: w1450 -> [w1451]
        stop <- FALSE stop-if-true
        n779 = flat-sequence {
          tunnel: w1459 -> [w1462]
          tunnel: [w1463] -> w1457
          tunnel: [w1462] -> w1455
          tunnel: [w1461] -> w1452
          tunnel: w1451 -> [w1461]
          tunnel: [w1466] -> w1458
          tunnel: w1457 -> [w1466]
          tunnel: [w1465] -> w1456
          tunnel: w1455 -> [w1465]
          tunnel: w1452 -> [w1464]
          tunnel: [w1475] -> w1454
          tunnel: w1458 -> [w1495]
          tunnel: w1456 -> [w1492]
          tunnel: [w1484] -> w1453
          frame #0 {
            n780 = call "Loop Timer14"("Count(Ticks)"=w1462) -> ("Tick Count(Ticks)"=w1463:u16)
          }
          frame #1 {
            n781 = xnode "FPGA I/O Node"("Connector1/DIO28"=w1464) -> ()  [unwired: 1 in, 1 out]
          }
          frame #2 {
            n782 = feedback-in #66(w1495) -> ()
            n783 = feedback #66(w1495) -> (w1494:u16)
            n784 = Subtract(x=w1495, y=w1494) -> (x-y=w1493:u16)
            n785 = Subtract(x=w1493, y=w1492) -> (x-y=w1468:u16)
            n786 = Number To Boolean Array(number=w1468) -> (Boolean array=w1469:bool[])
            n787 = Or Array Elements(Boolean array=w1469) -> (logical OR=w1467:bool)
            n788 = Boolean To (0,1)(Boolean="+ phase (BI D)") -> (0, 1=w1480:i16)
            n789 = Multiply(x=w1480, y="Phase count adjustment (BI D)") -> (x*y=w1477:i16)
            n790 = Boolean To (0,1)(Boolean=w1467) -> (0, 1=w1474:i16)
            n791 = To Unsigned Byte Integer(number=w1474) -> (unsigned 8bit integer=w1471:u8)
            n792 = feedback #67(i16 0) -> (w1478:i16)
            n793 = feedback #68(u8 0) -> (w1472:u8)
            n794 = Add(x=w1471, y=w1472) -> (x+y=w1470:u8)
            "Blue Late Counter (D)" <- w1470
            n795 = feedback-in #68(w1470) -> ()
            n796 = Subtract(x=w1478, y=w1477) -> (x-y=w1476:i16)
            "BI Relative phase (D)" <- w1476
            n797 = feedback-in #67(w1476) -> ()
            n798 = feedback #69(TRUE) -> (w1487:bool)
            n799 = case shown="2" "Blue Laser Operating Mode (D)" {
              tunnel: [TRUE FALSE w1501] -> w1484
              tunnel: w1487 -> [_ _ w1498]
              frame 0, Default {
              }
              frame 1 {
              }
              frame 2 {
                n800 = Not(x=w1498) -> (.not. x?=w1500:bool)
                n801 = Select(t=w1500, s="Invert BI (D)", f=w1498) -> (s? t:f=w1501:bool)
              }
            }
            n802 = Not(x=w1487) -> (.not. x?=w1483:bool)
            n803 = Select(t="Blue interlace ON count (D)", s=w1483, f="Blue interlace OFF count (D)") -> (s? t:f=w1489:u16)
            n804 = Subtract(x=w1489, y=w1468) -> (x-y=w1481:u16)
            n805 = Add(x=w1481, y=w1477) -> (x+y=w1475:u16)
            n806 = feedback-in #69(w1483) -> ()
          }
        }
      }
    }
    frame Enabled {
    }
  }
